vi "Measurement.vi"(0 "Position":T3(array[cluster]) {"Z" format="%.1f"; "Y" format="%.1f"; "X" format="%.1f"}, 1 "setup":T4=enum."Show Setup", 2 "Post Process":T2, 4 "File":T5, 5 "Results file":path, 7 "Raw data file":path, 11 "Setup filename":string) -> (14 "2nd plot":cluster{"X array":dbl[], "Y array":dbl[]}[](graph), 19 "Status Out":T1)   [LabVIEW 2015]
uses:
  Anemometry Sub Vis/Controls/Save_Data.ctl
  Anemometry Sub Vis/Controls/Setup.ctl
  Anemometry Sub Vis/Controls/Graph_Type.ctl
  Anemometry Sub Vis/Controls/Post_Process.ctl
  Anemometry Sub Vis/Gen Trav/Multi_Run_Status.ctl
  Anemometry Sub Vis/Controls/Inst_type.ctl
  ADAM Client/Sub VIs/ADAM Controls/Traverse_Level_State.ctl
  Anemometry Sub Vis/File/Setup_Filetype.ctl
  Anemometry Sub Vis/Globals/Meas_global.vi
  Anemometry Sub Vis/Globals/Trav_pos_global.vi
  Anemometry Sub Vis/Globals/Plug_in_data_global.vi
  Anemometry Sub Vis/Globals/Dynamic_call_global.ph.vi
  Anemometry Sub Vis/Globals/Preference_global.vi
  Anemometry Sub Vis/Globals/Constants_global.vi
  Anemometry Sub Vis/Globals/LDA_meas_global_2.vi
  Anemometry Sub Vis/Globals/LDA_meas_global_1.vi
  Anemometry Sub Vis/Acquisition/PWA/PWAtasksGLOBAL.vi
  Anemometry Sub Vis/Acquisition/Data_Translation/DataTranslation_global.vi
  Anemometry Sub Vis/Globals/Gas_management_global.vi
panel:
  in  "PP next block":bool
  out "Pause message":string
  out "Statistics":string[][](table)
  out "Actual Sampling freq":dbl=100.0 format="%.1f"
  in  "Desired Sampling freq (Hz)":dbl=100.0 format="%.1f"
  out "Current Block No":i32=5 caption="Current Block"
  in  "Pause":bool
  in  "No of Blocks":i32=5
  in  "stop":bool
  in  "No of samples":i32=1000 min=0 step=1
  in  "Tab Control":T6(tab)
  in  "Second Graph":T8={"Plot 1"=2, "Plot 2"=1, "Save graph"=0, "Plot Type"=enum."Vel histogram"} {"Save graph" items=["Do not save plot", "Save plot"]; "Plot 2" items=["Nothing", "mm"]; "Plot 1" items=["Nothing", "mm"]}
  in  "First Graph":T8={"Plot 1"=1, "Plot 2"=2, "Save graph"=0, "Plot Type"=enum."Velocity trace"} {"Save graph" items=["Do not save plot", "Save plot"]; "Plot 2" items=["Nothing", "mm"]; "Plot 1" items=["Nothing", "mm"]}
  out "First plot":cluster{"X array":dbl[], "Y array":dbl[]}[](graph)
  in  "Comments":string
  out "uv":dbl[][](graph)=[[-0.041806189081711534, -0.046435429052714985, -0.04035660097427599, -0.042187605126076694, -0.042052555599004206]]
  out "u^4":dbl[][](graph)
  out "u^3":dbl[][](graph)
  out "u^2":dbl[][](graph)=[[0.09743628875280319, 0.10575821456272283, 0.10126262927293661, 0.09890442087602569, 0.1022948212436432]]
  out "U":dbl[][](graph)=[[0.8295029456391334, 0.8915896983798417, 0.8415763502225625, 0.8394746126219594, 0.8466062785395404]]
  in  "Block average display control":cluster{"Name":string, "Include":bool}[](array[cluster])=[{"Name"="FF (C)", "Include"=FALSE}]
  in  "No of bins in histogram":i32=100
  out "Measurement time (min)":dbl=6.0 format="%.2f"
  in  "Correlate?":T9(ring)
  out "Diagnostic info":string[][](table)
  out "Array U":dbl[][](array[numeric]) format="%.2e"
  out "Array u^2":dbl[][](array[numeric]) format="%.2e"
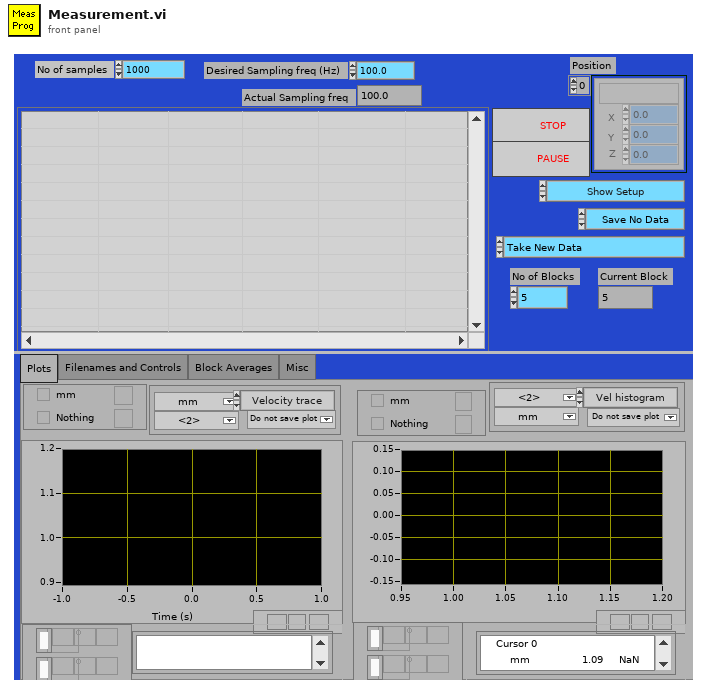
[diagram p1: front panel]
types:
  T1 = typedef "Multi_Run_Status.ctl" = enum16{"Continue", "Jump to Next Point", "Jump to Next Row", "Jump To Fall Back", "Terminate Run"}
  T2 = typedef "Post_Process.ctl" = enum16{"Take New Data", "Post Process Raw Data File"}
  T3 = cluster{"Name":string, "X":dbl, "Y":dbl, "Z":dbl}[]
  T4 = typedef "Setup.ctl" = enum16{"Run Program", "Show Setup", "Save Current Setup", "Setup Front Panel"}
  T5 = typedef "Save_Data.ctl" = enum16{"Save No Data", "Save Data"}
  T6 = enum32{"Plots", "Filenames and Controls", "Block Averages", "Misc"}
  T7 = typedef "Graph_Type.ctl" = enum16{"Show no graph", "Voltage trace", "Velocity trace", "Vel histogram", "Spectrum", "f.E(f) v Log f", "Auto-Corr"}
  T8 = cluster{"Plot 1":u16, "Plot 2":u16, "Save graph":u16, "Plot Type":T7}
  T9 = enum16{"Cross correlation off", "Show correlation panel", "Correlate without activating panel"}
  T10 = enum32{"Bad", "Idle", "Run top level", "Running"}
  T11 = cluster{"Name":string, "X":dbl, "Y":dbl, "Z":dbl}
  T12 = enum16{"Velocity", "Transit time", "Arrival time"}
  T13 = enum16{"Save no data", "Save data in new files", "Save data in existing files"}
  T14 = typedef "Inst_type.ctl" = enum16{"Propeller anemometer", "Raw voltage", "Pressure Transducer", "Pitot-static tube", "Preston tube", "Hot wire", "Cross wire 1", "Cross wire 2", "Generic Linear", "Generic Polynomial", "Generic BackPoly", "Fast FID", "Thermocouple", "Cold wire", "Pulsed Wire", "LDA Vel", "LDA Tran time", "LDA Arr time", "Microphone"}
  T15 = enum16{"Zero or one", "One", "Zero or more", "One or more"}
  T16 = cluster{"Weighting":dbl[], "Time (ms)":dbl[], "Voltage":dbl[], "Eng Values":dbl[]}
  T17 = typedef "Traverse_Level_State.ctl" = enum16{"Running", "Complete"}
  T18 = typedef "Setup_Filetype.ctl" = enum16{"Measurement Setups", "Calibration Setups", "General", "Results File Plotter Setups", "Speed Calib Tweaks"}
  T19 = typedef "Analysis_info_cluster.ctl" = cluster{"Colour":u32, "Inst type":T14, "Inst name":string, "Symbol":string, "Code name":string, "Extra Info":string, "Inst Array":T20, "Extra Titles":string[], "Extra Values":string[], "U":dbl, "u^2":dbl, "u^3":dbl, "u^4":dbl, "Skew_u":dbl, "Kurt_u":dbl, "Sd Error in Mean":dbl, "% u'/U":dbl, "X":dbl, "Y":dbl, "Z":dbl, "Timescale integral to 25%":dbl, "Sd Error in Variance":dbl, "Calib File":path, "Calib Constants":dbl[], "Output Position":bool, "Full Stats":bool, "Av Sampling Rate":dbl, "Av No of Samples":dbl, "Total Meas Time (s)":dbl, "ADAM Ch Name":string, "Max value":dbl, "Min value":dbl}
  T20 = typedef "Instrument_Array.ctl" = enum16{"PWA", "LDA", "Analogue"}
  T21 = typedef "LDA_Setup.ctl" = cluster{"dimensions":enum16{"1D", "2D"}, "Analogue Freq Multiplier":dbl}
  T22 = enum16{"Velocity", "Transit time", "Arrival time"}[]
  T23 = typedef "BSA_Type.ctl" = enum16{"57N11", "BSA F60"}
  T24 = typedef "BSA_info_Cluster.ctl" = cluster{"GPIB Address":string, "No of Check Bytes":i32, "Extra Info":string, "COLOUR":u32, "Wavelength (nm)":dbl}
  T25 = typedef "Ch_and_Spans.ctl" = cluster{"high limit (10V)":sgl, "low limit (-10V)":sgl, "Ch No":i16, "Var name":string, "Use Latest Calib":bool}
  T26 = cluster{"Weighting":dbl[], "Time (ms)":dbl[], "Voltage":dbl[], "Eng Values":dbl[]}[]
  T27 = cluster{"Insts for plotting[0]":u16, "Insts for plotting[1]":u16}
  T28 = typedef "PWA_Data.ctl" = enum16{"No PWA Data", "One Ch PWA"}
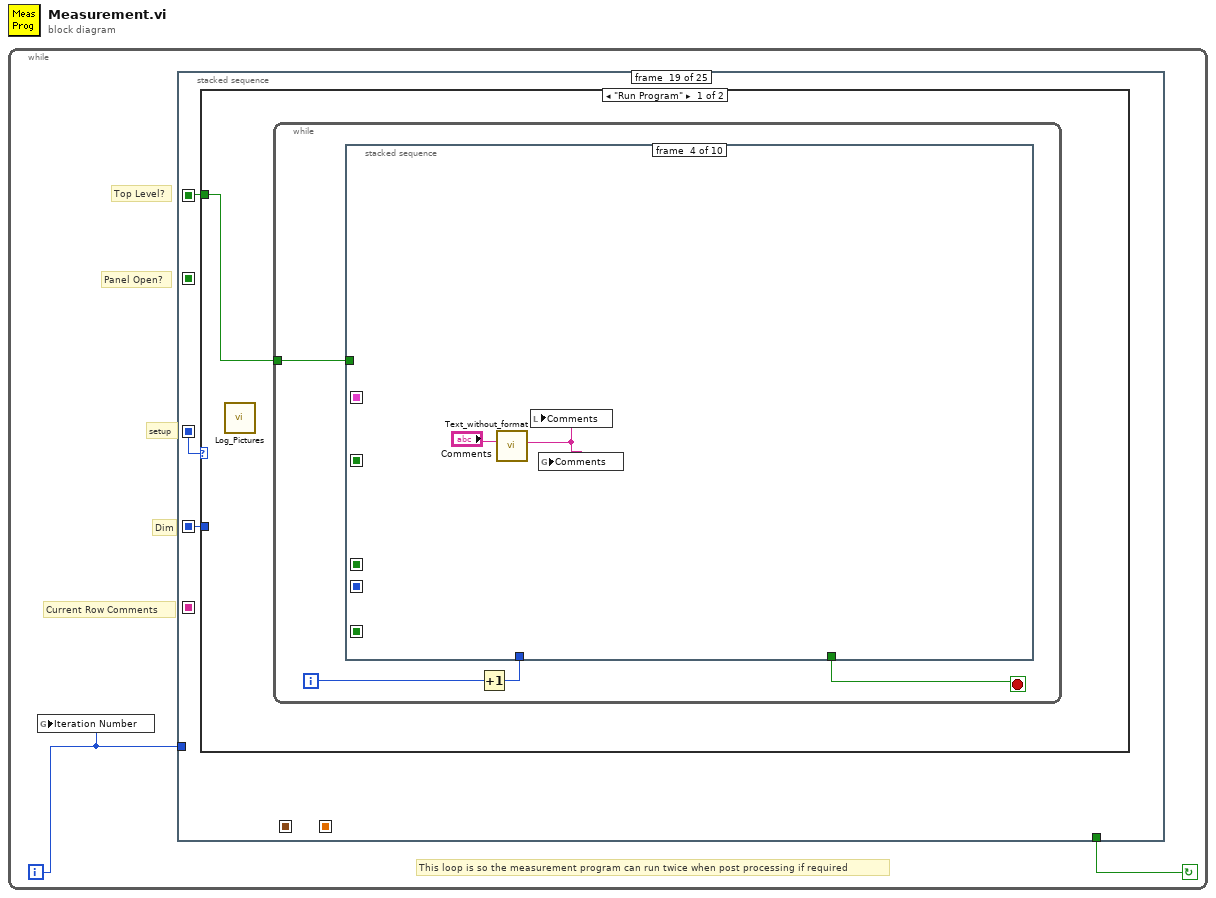
[diagram p0: block diagram]
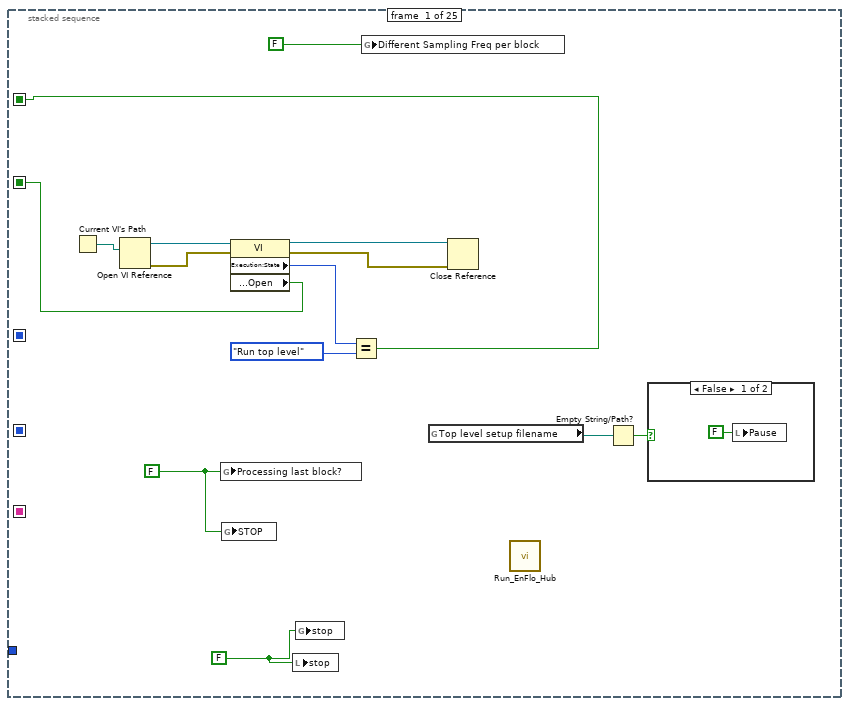
[diagram p2: hidden frame]
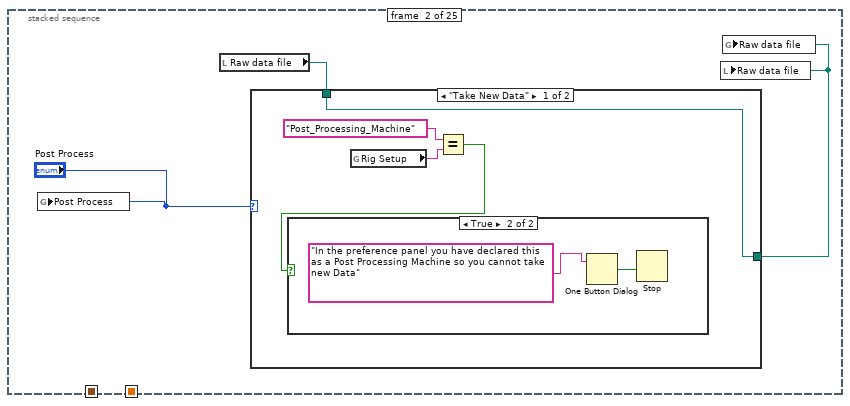
[diagram p4: hidden frame]
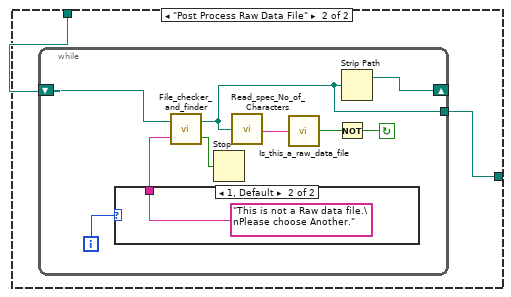
[diagram p6: hidden frame]
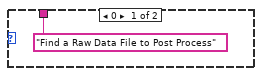
[diagram p7: hidden frame]
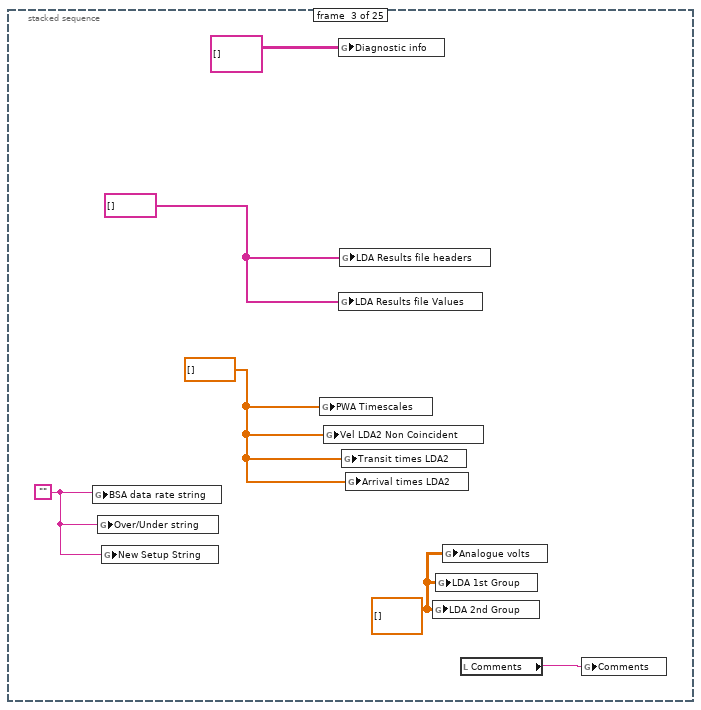
[diagram p8: hidden frame]
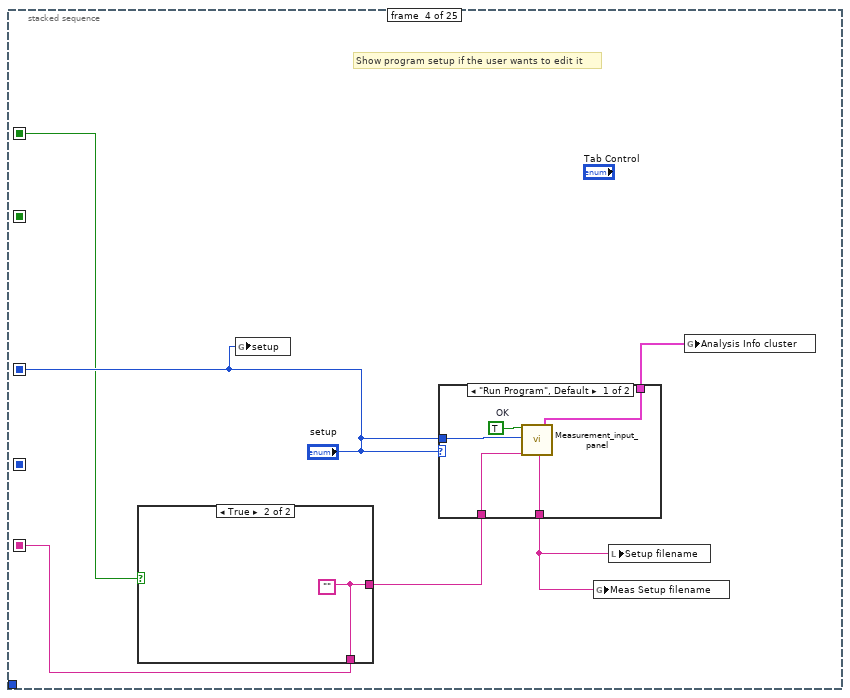
[diagram p9: hidden frame]
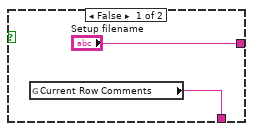
[diagram p10: hidden frame]
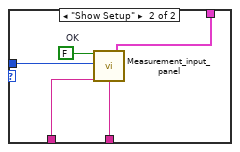
[diagram p11: hidden frame]
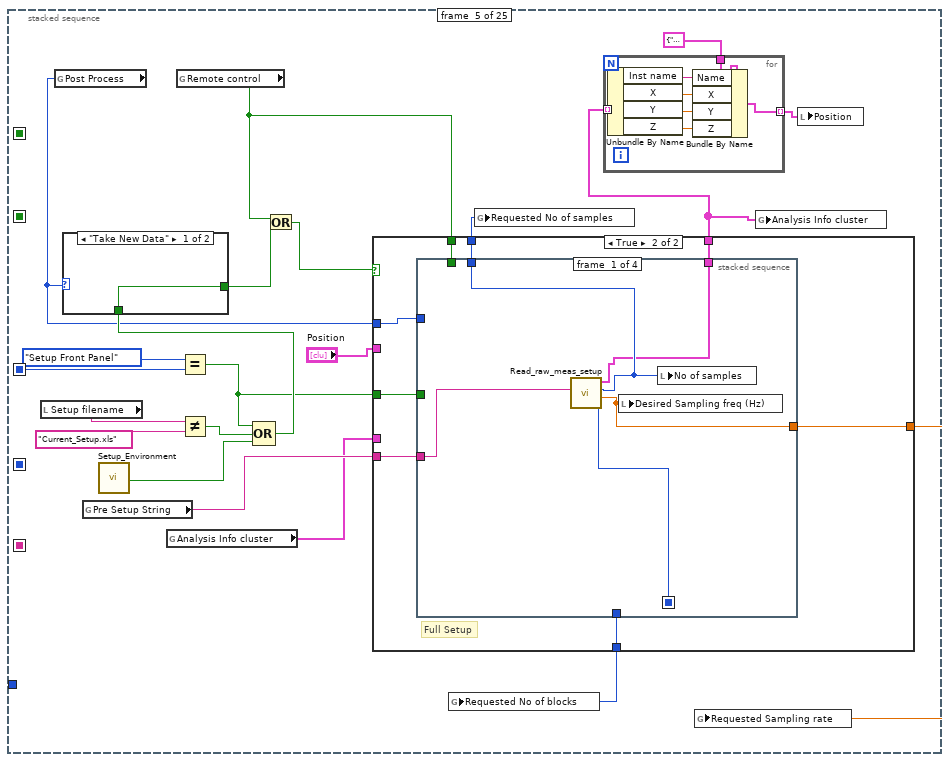
[diagram p12: hidden frame]
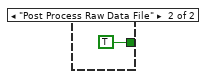
[diagram p13: hidden frame]
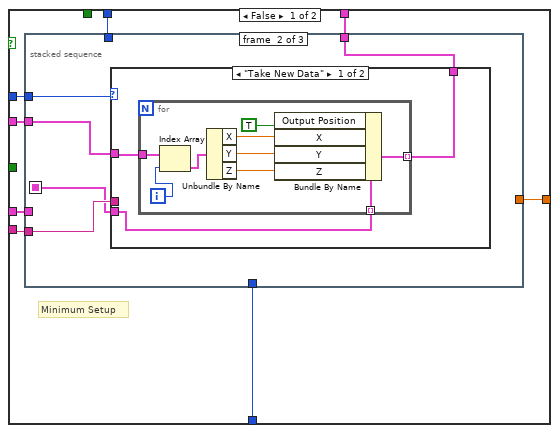
[diagram p14: hidden frame]
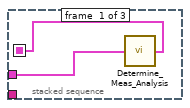
[diagram p15: hidden frame]
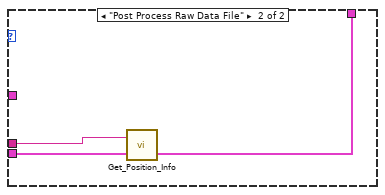
[diagram p16: hidden frame]
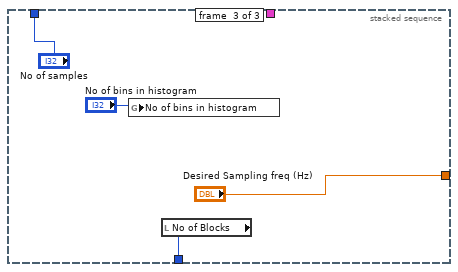
[diagram p17: hidden frame]
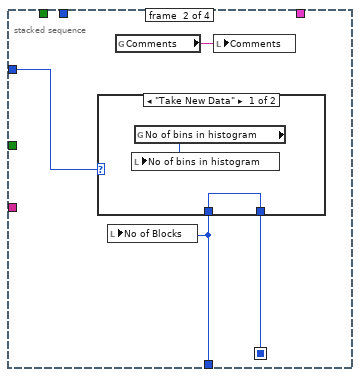
[diagram p18: hidden frame]
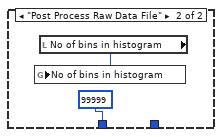
[diagram p19: hidden frame]
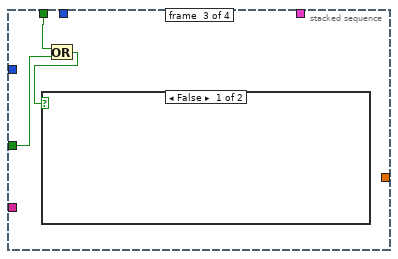
[diagram p20: hidden frame]
diagram:
  n1 = while {
    i -> [w1]
    stop <- w2 continue-if-true
    # "Current Row Comments"
    # "This loop is so the measurement program can run twice when post processing if required"
    # "Panel Open?"
    # "Top Level?"
    # "setup"
    # "Dim"
    n2 = global write "Meas_global.vi" "Iteration Number"(w1) -> ()
    n3 = stacked-sequence {
      seq-local: [_ _ _ _ _ _ _ _ w220 _ _ _ _ _ _ _ _ _ _ _ _ _ _ _ _] -> [_ _ _ _ _ _ _ _ _ _ _ _ _ _ _ _ _ _ w846 _ _ _ _ _ _]
      seq-local: [_ _ _ "setup" _ _ _ _ _ _ _ _ _ _ _ _ _ _ _ _ _ _ _ _ _] -> [_ _ _ _ w77 _ w184 _ w219 w308 _ _ _ _ w730 w749 w756 _ w847 w1047 w1097 w1167 _ _ w1288]
      seq-local: [_ _ _ _ _ _ _ _ _ _ _ _ _ _ _ _ w753 _ _ _ _ _ _ _ _] -> [_ _ _ _ _ _ _ _ _ _ _ _ _ _ _ _ _ _ _ w1037 _ _ _ _ _]
      seq-local: [w7 _ _ _ _ _ _ _ _ _ _ _ _ _ _ _ _ _ _ _ _ _ _ _ _] -> [_ _ _ w47 _ _ _ _ _ w288 _ _ _ _ w727 _ _ _ w845 _ _ _ _ _ _]
      seq-local: [w6 _ _ _ _ _ _ _ _ _ _ _ _ _ _ _ _ _ _ _ _ _ _ _ _] -> [_ _ _ _ _ _ _ _ _ _ _ _ w521 _ _ _ _ _ _ _ _ _ _ _ _]
      seq-local: [_ _ _ _ _ _ _ _ _ _ _ _ _ _ _ _ w751 _ _ _ _ _ _ _ _] -> [_ _ _ _ _ _ _ _ _ _ _ _ _ _ _ _ _ _ _ _ _ _ _ _ _]
      seq-local: [_ _ _ w46 _ _ _ _ _ _ _ _ _ _ _ _ _ _ _ _ _ _ _ _ _] -> [_ _ _ _ _ _ _ w215 _ _ _ _ _ _ _ _ _ _ _ _ _ _ _ w1251 _]
      tunnel: w1 -> [_ _ _ _ _ _ _ _ _ _ _ _ _ _ _ _ _ _ _ _ _ _ _ w1253 _]
      tunnel: [_ _ _ _ _ _ _ _ _ _ _ _ _ _ _ _ _ _ _ _ _ _ _ w1252 _] -> w2
      frame #0 {
        w15 = FALSE ("Processing last block?")
        w16 = FALSE ("stop")
        n4 = Current VI's Path() -> (path=w8:path)
        n5 = Open VI Reference(vi path=w8) -> (vi reference=w9:refnum<vi>, error out=w10:errorcluster)  [unwired: 1 in, 4 out]
        n6 = global write "Meas_global.vi" "Processing last block?"(w15) -> ()
        n7 = global write "PWAtasksGLOBAL.vi" "STOP"(w15) -> ()
        n8 = property class="VI"(reference=w9, error in=w10) -> (reference out=w11:refnum<vi>, error out=w12:errorcluster, "Execution:State"=w13:T10, "Front Panel.Open"=w6:bool)
        n9 = local write "stop"(w16) -> ()
        n10 = global write "Meas_global.vi" "stop"(w16) -> ()
        n11 = Equal?(x=w13, y=T10."Run top level" ("Exec.State")) -> (x = y?=w7:bool)
        n12 = global write "DataTranslation_global.vi" "Different Sampling Freq per block"(FALSE ("Different Sampling Freq per block")) -> ()
        n13 = global read "Trav_pos_global.vi" "Top level setup filename"() -> (w4:path)
        n14 = Close Reference(reference=w11, error in (no error)=w12) -> ()  [unwired: 1 out]
        n15 = call "Run_EnFlo_Hub.vi"() -> ()  [unwired: 1 in, 7 out]
        n16 = Empty String/Path?(string/path=w4) -> (empty?=w3:bool)
        n17 = case shown="False" w3 {
          frame False {
            n18 = local write "Pause"(FALSE ("Pause")) -> ()
          }
          frame True {
          }
        }
      }
      frame #1 {
        n19 = global write "Meas_global.vi" "Post Process"("Post Process") -> ()
        n20 = local read "Raw data file"() -> (w20:path)
        n21 = case shown="\"Take New Data\"" "Post Process" {
          tunnel: [w24 w28] -> w19
          tunnel: w20 -> [w24 w27]
          frame "Take New Data" {
            n22 = global read "Preference_global.vi" "Rig Setup"() -> (w23:string)
            n23 = Equal?(x="Post_Processing_Machine" ("Rig Setup"), y=w23) -> (x = y?=w21:bool)
            n24 = case shown="True" w21 {
              frame False {
              }
              frame True {
                n25 = One Button Dialog(message="In the preference panel you have declared this as a Post Processing Machine so you cannot take new Data") -> (true=w25:bool)  [unwired: 1 in]
                n26 = Stop(stop? (T)=w25) -> ()
              }
            }
          }
          frame "Post Process Raw Data File" {
            n27 = while {
              tunnel: [w30] -> w28
              shift-left: w27 -> [w32]
              shift-right: [w31] -> _
              i -> [w33]
              stop <- w34 continue-if-true
              n28 = case shown="1, Default" w33 {
                tunnel: ["Find a Raw Data File to Post Process" ("Promp if not found") "This is not a Raw data file.\nPlease choose Another." ("Promp if not found")] -> w37
                frame 0 {
                }
                frame 1, Default {
                }
              }
              n29 = call "File_checker_and_finder.vi"("Promp if not found"=w37, "Filename In"=w32) -> ("cancelled"=w29:bool, "Filename Out"=w30:path)
              n30 = Stop(stop? (T)=w29) -> ()
              n31 = call "Read_spec_No_of_Characters.vi"("Filename"=w30) -> ("character string"=w36:string)  [unwired: 1 out]
              n32 = call "Is_this_a_raw_data_file.vi"("character string"=w36) -> ("Raw Dat File?"=w35:bool)  [unwired: 2 out]
              n33 = Not(x=w35) -> (.not. x?=w34:bool)
              n34 = Strip Path(path=w30) -> (stripped path=w31:path)  [unwired: 1 out]
            }
          }
        }
        n35 = local write "Raw data file"(w19) -> ()
        n36 = global write "Meas_global.vi" "Raw data file"(w19) -> ()
      }
      frame #2 {
        w40 = dbl[][] [] ("LDA 2nd Group")
        w41 = dbl[] [] ("LDA Timescales")
        w43 = string[] [] ("Plug in values")
        w45 = ""
        n37 = global write "Meas_global.vi" "BSA data rate string"(w45) -> ()
        n38 = global write "Meas_global.vi" "Over/Under string"(w45) -> ()
        n39 = global write "Meas_global.vi" "New Setup String"(w45) -> ()
        n40 = global write "PWAtasksGLOBAL.vi" "PWA Timescales"(w41) -> ()
        n41 = global write "LDA_meas_global_2.vi" "Vel LDA2 Non Coincident"(w41) -> ()
        n42 = global write "Meas_global.vi" "Diagnostic info"(string[][] [] ("Diagnostic info")) -> ()
        n43 = global write "LDA_meas_global_1.vi" "LDA Results file Values"(w43) -> ()
        n44 = global write "LDA_meas_global_1.vi" "LDA Results file headers"(w43) -> ()
        n45 = global write "LDA_meas_global_2.vi" "Transit times LDA2"(w41) -> ()
        n46 = global write "LDA_meas_global_2.vi" "Arrival times LDA2"(w41) -> ()
        n47 = global write "LDA_meas_global_2.vi" "LDA 2nd Group"(w40) -> ()
        n48 = global write "LDA_meas_global_2.vi" "LDA 1st Group"(w40) -> ()
        n49 = global write "Meas_global.vi" "Analogue volts"(w40) -> ()
        n50 = local read "Comments"() -> (w44:string)
        n51 = global write "Meas_global.vi" "Comments"(w44) -> ()
      }
      frame #3 {
        # "Show program setup if the user wants to edit it"
        n52 = case shown="True" w47 {
          tunnel: ["Setup filename" w54] -> w50
          tunnel: [w52 w54] -> w46
          frame False {
            n53 = global read "Meas_global.vi" "Current Row Comments"() -> (w52:string)
          }
          frame True {
            w54 = ""
          }
        }
        n54 = global write "Meas_global.vi" "setup"("setup") -> ()
        n55 = case shown="\"Run Program\", Default" "setup" {
          tunnel: [w58 w63] -> w51
          tunnel: w50 -> [w57 w62]
          tunnel: [w56 w61] -> w49
          tunnel: "setup" -> [w55 w60]
          frame "Run Program", Default {
            w59 = TRUE  # OK
            n56 = call "Measurement_input_panel.vi"("OK"=w59, "setup"=w55, "Setup filename"=w57) -> ("Setup filename out"=w56:string, "Analysis Info cluster"=w58:T19[])  [unwired: 15 out]
          }
          frame "Show Setup" {
            w64 = FALSE  # OK
            n57 = call "Measurement_input_panel.vi"("OK"=w64, "setup"=w60, "Setup filename"=w62) -> ("Setup filename out"=w61:string, "Analysis Info cluster"=w63:T19[])  [unwired: 15 out]
          }
        }
        n58 = global write "Meas_global.vi" "Meas Setup filename"(w49) -> ()
        n59 = local write "Setup filename"(w49) -> ()
        n60 = global write "Meas_global.vi" "Analysis Info cluster"(w51) -> ()
      }
      frame #4 {
        n61 = local read "Setup filename"() -> (w81:string)
        n62 = global read "Meas_global.vi" "Post Process"() -> (w76:T2)
        n63 = global read "Meas_global.vi" "Pre Setup String"() -> (w72:string)
        n64 = call "Setup_Environment.vi"() -> ("First Time"=w73:bool)  [unwired: 1 in]
        n65 = global read "Meas_global.vi" "Analysis Info cluster"() -> (w69:T19[])
        n66 = global read "Meas_global.vi" "Remote control"() -> (w71:bool)
        n67 = Equal?(x=Setup."Setup Front Panel" ("setup"), y=w77) -> (x = y?=w70:bool)
        n68 = Not Equal?(x=w81, y="Current_Setup.xls" ("Setup filename")) -> (x != y?=w79:bool)
        n69 = Compound Arithmetic op=OR(w70, w79, w73) -> (w78:bool)
        n70 = case shown="\"Take New Data\"" w76 {
          tunnel: [w93 TRUE] -> w85
          tunnel: w78 -> [w93 _]
          frame "Take New Data" {
          }
          frame "Post Process Raw Data File" {
          }
        }
        n71 = Or(x=w71, y=w85) -> (x .or. y?=w84:bool)
        n72 = case shown="True" w84 {
          tunnel: w76 -> [w98 w136]
          tunnel: [w102 w135] -> w74
          tunnel: [w101 w130] -> w83
          tunnel: [w100 w134] -> w82
          tunnel: [w99 w133] -> w68
          tunnel: w72 -> [w97 w132]
          tunnel: "Position" -> [w96 _]
          tunnel: w71 -> [_ w131]
          tunnel: w70 -> [_ w129]
          tunnel: w69 -> [w95 _]
          frame False {
            # "Minimum Setup"
            n73 = stacked-sequence {
              seq-local: [w103 _ _] -> [_ w105 _]
              tunnel: [_ _ "Desired Sampling freq (Hz)"] -> w102
              tunnel: [_ _ w127] -> w101
              tunnel: [_ _ "No of samples"] -> w100
              tunnel: [_ w108 _] -> w99
              tunnel: w98 -> [_ w109 _]
              tunnel: w97 -> [_ w107 _]
              tunnel: w96 -> [_ w106 _]
              tunnel: w95 -> [w104 _ _]
              frame #0 {
                n74 = call "Determine_Meas_Analysis.vi"("Analysis info Cluster In"=w104) -> ("Analysis info Cluster Out"=w103:T19[])
              }
              frame #1 {
                n75 = case shown="\"Take New Data\"" w109 {
                  tunnel: [w110 w122] -> w108
                  tunnel: w106 -> [w112 _]
                  tunnel: w107 -> [_ w123]
                  tunnel: w105 -> [w111 w124]
                  frame "Take New Data" {
                    n76 = for {
                      tunnel: w112 -> [w115]
                      tunnel: w111 -> [w121] mode=indexing
                      tunnel: [w117] -> w110 mode=indexing
                      i -> [w116]
                      n77 = Index Array(array=w115, index=w116) -> (element=w114:T11)
                      n78 = Unbundle By Name(w114) -> ("X"=w118:dbl, "Y"=w119:dbl, "Z"=w120:dbl)
                      n79 = Bundle By Name(cluster=w121, "Output Position"=TRUE, "X"=w118, "Y"=w119, "Z"=w120) -> (w117:T19)
                    }
                  }
                  frame "Post Process Raw Data File" {
                    n80 = call "Get_Position_Info.vi"("Analysis Info cluster"=w124, "Setup file string"=w123) -> ("Analysis Info cluster 2"=w122:T19[])  [unwired: 1 in]
                  }
                }
              }
              frame #2 {
                n81 = global write "Meas_global.vi" "No of bins in histogram"("No of bins in histogram") -> ()
                n82 = local read "No of Blocks"() -> (w127:i32)
              }
            }
          }
          frame True {
            # "Full Setup"
            n83 = stacked-sequence {
              seq-local: [w138 _ _ _] -> [_ w143 _ _]
              tunnel: w136 -> [_ w144 _ w159]
              tunnel: [w141 _ _ _] -> w135
              tunnel: [w140 _ _ _] -> w134
              tunnel: [w137 _ _ _] -> w133
              tunnel: w132 -> [w139 _ _ _]
              tunnel: w131 -> [_ _ w152 _]
              tunnel: [_ w142 _ _] -> w130
              tunnel: w129 -> [_ _ w151 _]
              frame #0 {
                n84 = call "Read_raw_meas_setup.vi"("Setup file string"=w139) -> ("No of Blocks"=w138:i32, "Sampling freq (Hz)"=w141:dbl, "No of samples"=w140:i32, "Analysis Info cluster 2"=w137:T19[])  [unwired: 5 out]
                n85 = local write "Desired Sampling freq (Hz)"(w141) -> ()
                n86 = local write "No of samples"(w140) -> ()
              }
              frame #1 {
                n87 = case shown="\"Take New Data\"" w144 {
                  tunnel: [w147 99999 ("No of Blocks")] -> w142
                  tunnel: w143 -> [w147 _]
                  frame "Take New Data" {
                    n88 = global read "Meas_global.vi" "No of bins in histogram"() -> (w146:i32)
                    n89 = local write "No of bins in histogram"(w146) -> ()
                  }
                  frame "Post Process Raw Data File" {
                    n90 = local read "No of bins in histogram"() -> (w148:i32)
                    n91 = global write "Meas_global.vi" "No of bins in histogram"(w148) -> ()
                  }
                }
                n92 = local write "No of Blocks"(w142) -> ()
                n93 = global read "Meas_global.vi" "Comments"() -> (w145:string)
                n94 = local write "Comments"(w145) -> ()
              }
              frame #2 {
                n95 = Or(x=w152, y=w151) -> (x .or. y?=w150:bool)
                n96 = case shown="False" w150 {
                  frame False {
                  }
                  frame True {
                    n97 = global read "Meas_global.vi" "Pre Setup String"() -> (w153:string)
                    n98 = call "Get_Characters_from_string.vi"("Input string"=w153, "Variable name"="Results filename") -> ("Status"=w156:enum16{"Char in string", "Char not in string"}, "Value"=w155:string)  [unwired: 1 in]
                    n99 = case shown="\"Char in string\"" w156 {
                      tunnel: w155 -> [w158 _]
                      frame "Char in string" {
                        n100 = String To Path(string=w158) -> (path=w157:path)
                        n101 = local write "Results file"(w157) -> ()
                      }
                      frame "Char not in string" {
                      }
                    }
                  }
                }
              }
              frame #3 {
                n102 = case shown="\"Post Process Raw Data File\"" w159 {
                  frame "Take New Data" {
                    n103 = global read "Meas_global.vi" "Second Graph"() -> (w160:T8)
                    n104 = global read "Meas_global.vi" "First Graph"() -> (w161:T8)
                    n105 = local write "Second Graph"(w160) -> ()
                    n106 = local write "First Graph"(w161) -> ()
                  }
                  frame "Post Process Raw Data File" {
                  }
                }
              }
            }
          }
        }
        n107 = global write "Meas_global.vi" "Requested No of blocks"(w83) -> ()
        n108 = global write "Meas_global.vi" "Requested No of samples"(w82) -> ()
        n109 = for {
          tunnel: w68 -> [w92] mode=indexing
          tunnel: [w88] -> w66 mode=indexing
          tunnel: T11 {"Name"="", "X"=0.0, "Y"=0.0, "Z"=0.0} ("Position") -> [w87]
          n110 = Unbundle By Name(w92) -> ("Inst name"=w86:string, "X"=w89:dbl, "Y"=w90:dbl, "Z"=w91:dbl)
          n111 = Bundle By Name(cluster=w87, "Name"=w86, "X"=w89, "Y"=w90, "Z"=w91) -> (w88:T11)
        }
        n112 = global write "Meas_global.vi" "Requested Sampling rate"(w74) -> ()
        n113 = global write "Meas_global.vi" "Analysis Info cluster"(w68) -> ()
        n114 = local write "Position"(w66) -> ()
      }
      frame #5 {
        n115 = global read "Meas_global.vi" "Post Process"() -> (w162:T2)
        n116 = case shown="\"Post Process Raw Data File\"" w162 {
          tunnel: [w165 w166] -> w163
          frame "Take New Data" {
            n117 = Get Date/Time In Seconds() -> (seconds since 1Jan1904=w164:timestamp)
            n118 = To Double Precision Float(number=w164) -> (double precision float=w165:dbl)
          }
          frame "Post Process Raw Data File" {
            n119 = global read "Meas_global.vi" "Pre Setup String"() -> (w169:string)
            n120 = call "Get_Characters_from_string.vi"("Input string"=w169, "Variable name"="Seconds since 1/1/04") -> ("Value"=w167:string)  [unwired: 1 in, 1 out]
            n121 = call "String_2_Number.vi"("Value"=w167) -> ("Numeric"=w166:dbl)
          }
        }
        n122 = global write "Meas_global.vi" "Time Data was Aquired"(w163) -> ()
      }
      frame #6 {
        n123 = global read "Dynamic_call_global.ph.vi" "Initial Plug Ins"() -> (w189:string[])
        n124 = global read "Trav_pos_global.vi" "Source Control?"() -> (w186:bool)
        n125 = local read "Setup filename"() -> (w177:string)
        n126 = global read "Meas_global.vi" "Post Process"() -> (w175:T2)
        n127 = global read "Preference_global.vi" "Rig Setup"() -> (w172:string)
        n128 = Search 1D Array(1D array=w189, element="Puff_using_Arduino.vi") -> (index of element=w187:i32)  [unwired: 1 in]
        n129 = Equal?(x=w172, y="EnFlo_Tunnel") -> (x = y?=w170:bool)
        n130 = Equal?(x=w175, y=Post_Process."Take New Data" ("Post Process")) -> (x = y?=w173:bool)
        n131 = Equal?(x=Setup."Run Program" ("setup"), y=w184) -> (x = y?=w182:bool)
        n132 = Less Than 0?(x=w187) -> (x < 0?=w179:bool)
        n133 = Not Equal?(x=w177, y="Meas_FF_Bkgnd_Setup.xls") -> (x != y?=w181:bool)
        n134 = Not Equal?(x=w177, y="Auto_Calib_Setup.xls") -> (x != y?=w176:bool)
        n135 = Compound Arithmetic op=AND(w186, w182, w181, w176, w173, w170) -> (w180:bool)
        n136 = case shown="True" w180 {
          tunnel: w179 -> [_ w190]
          frame False {
          }
          frame True {
            n137 = global read "Gas_management_global.vi" "Source Live"() -> (w191:bool)
            n138 = Not(x=w191) -> (.not. x?=w192:bool)
            n139 = Select(t=w191, s=w190, f=w192) -> (s? t:f=w193:bool)
            n140 = global read "Preference_global.vi" "Default Source Establishment Time (s)"() -> (w194:dbl)
            n141 = case shown="False" w193 {
              tunnel: w194 -> [w196 w209]
              tunnel: w190 -> [w195 _]
              frame False {
                n142 = stacked-sequence {
                  tunnel: w196 -> [_ w205]
                  tunnel: w195 -> [w197 _]
                  frame #0 {
                    n143 = case shown="False" w197 {
                      tunnel: [w202 w204] -> w199
                      tunnel: [w201 w203] -> w198
                      frame True {
                        w201 = u32 0  # Time to hold source OFF (microseconds)
                        w202 = u32 1  # Time to hold source ON (microseconds)
                      }
                      frame False {
                        w203 = u32 1  # Time to hold source OFF (microseconds)
                        w204 = u32 0  # Time to hold source ON (microseconds)
                      }
                    }
                    n144 = call "Arduino_Timed_Release.vi"("Time to hold source ON (microseconds)"=w199, "Time to hold source OFF (microseconds)"=w198, "Number of cycles"=u16 1) -> ()  [unwired: 2 out]
                  }
                  frame #1 {
                    n145 = Greater Than 0?(x=w205) -> (x > 0?=w206:bool)
                    n146 = case shown="True" w206 {
                      tunnel: w205 -> [_ w207]
                      frame False {
                      }
                      frame True {
                        n147 = call "Wait_Seconds_with_display.vi"("Message"="Est Source", "Seconds to wait"=w207) -> ()  [unwired: 2 out]
                      }
                    }
                  }
                }
              }
              frame True {
                n148 = global read "Gas_management_global.vi" "Source Live Last changed"() -> (w213:timestamp)
                n149 = Get Date/Time In Seconds() -> (seconds since 1Jan1904=w214:timestamp)
                n150 = Subtract(x=w214, y=w213) -> (x-y=w212:dbl)
                n151 = Subtract(x=w209, y=w212) -> (x-y=w210:dbl)
                n152 = call "Wait_Seconds_with_display.vi"("Message"="Est Source", "Seconds to wait"=w210) -> ()  [unwired: 2 out]
              }
            }
          }
        }
      }
      frame #7 {
        n153 = local read "Comments"() -> (w218:string)
        n154 = Concatenate Strings(w215, w218) -> (w217:string)
        n155 = call "Text_without_format.vi"("Input string"=w217) -> ("Output string"=w216:string)
        n156 = local write "Comments"(w216) -> ()
        n157 = global write "Meas_global.vi" "Comments"(w216) -> ()
      }
      frame #8 {
        n158 = global read "Meas_global.vi" "LDA set up"() -> (w221:T21)
        n159 = Unbundle By Name(w221) -> ("dimensions"=w220:enum16{"1D", "2D"})
        n160 = global read "Meas_global.vi" "LDA data"() -> (w228:enum16{"No LDA data", "Take LDA data"})
        n161 = global read "Meas_global.vi" "Post Process"() -> (w230:T2)
        n162 = Equal?(x=w219, y=Setup."Show Setup" ("setup")) -> (x = y?=w222:bool)
        n163 = Equal?(x=w228, y=enum16{"No LDA data", "Take LDA data"}."Take LDA data" ("LDA data")) -> (x = y?=w224:bool)
        n164 = Equal?(x=w230, y=Post_Process."Take New Data" ("Post Process")) -> (x = y?=w225:bool)
        n165 = Compound Arithmetic op=AND(w224, w225) -> (w223:bool)
        n166 = case shown="True" w223 {
          tunnel: w220 -> [_ w239]
          tunnel: w219 -> [_ w238]
          tunnel: w222 -> [_ w236]
          frame False {
            n167 = Build Array(T12."Velocity", T12."Transit time", T12."Arrival time") -> (w231:T22)
            n168 = global write "LDA_meas_global_1.vi" "Number of measured quantities"(3 ("Number of measured quantities")) -> ()
            n169 = global write "LDA_meas_global_2.vi" "data type"(w231) -> ()
            n170 = global write "LDA_meas_global_1.vi" "data type"(w231) -> ()
          }
          frame True {
            n171 = global read "LDA_meas_global_1.vi" "BSA Type"() -> (w237:T23)
            n172 = case shown="\"BSA F60\"" w237 {
              tunnel: w239 -> [w241 _]
              tunnel: w238 -> [w240 _]
              tunnel: w236 -> [_ w277]
              frame "57N11" {
                n173 = stacked-sequence {
                  tunnel: w241 -> [w244 w270]
                  tunnel: w240 -> [w243 _]
                  frame #0 {
                    n174 = global read "Meas_global.vi" "Remote control"() -> (w242:bool)
                    n175 = case shown="\"1D\"" w244 {
                      tunnel: w243 -> [w246 w259]
                      tunnel: w242 -> [w245 w258]
                      frame "2D" {
                        n176 = while {
                          tunnel: w245 -> [w247]
                          tunnel: w246 -> [w248]
                          stop <- w249 continue-if-true
                          n177 = stacked-sequence {
                            tunnel: [_ _ w255] -> w249
                            tunnel: w248 -> [w250 w252 _]
                            tunnel: w247 -> [_ _ w254]
                            frame #0 {
                              w251 = "1"  # BSA Number
                              n178 = call "Control_BSA_setup.vi"("setup"=w250, "BSA number"=w251) -> ()  [unwired: 14 out]
                            }
                            frame #1 {
                              w253 = "2"  # BSA Number
                              n179 = call "Control_BSA_setup.vi"("setup"=w252, "BSA number"=w253) -> ()  [unwired: 14 out]
                            }
                            frame #2 {
                              n180 = case shown="False" w254 {
                                tunnel: [w256 FALSE ("ok")] -> w255
                                frame False {
                                n181 = call "BSA_setup_check.vi"() -> ("ok"=w256:bool)
                                }
                                frame True {
                                }
                              }
                            }
                          }
                        }
                      }
                      frame "1D" {
                        n182 = stacked-sequence {
                          tunnel: w259 -> [w260 _]
                          tunnel: w258 -> [_ _]
                          frame #0 {
                            w261 = "1"  # BSA Number
                            n183 = call "Control_BSA_setup.vi"("setup"=w260, "BSA number"=w261) -> ()  [unwired: 14 out]
                          }
                          frame #1 {
                            n184 = global read "LDA_meas_global_2.vi" "BSA2 info"() -> (w262:T24)
                            n185 = Unbundle By Name(w262) -> ("GPIB Address"=w263:string)
                            n186 = call "Set_BSA_Coincidence.vi"("GPIB address"=w263, "Set Coincidence"=enum16{"Slave", "Master", "Private"}."Slave") -> ()  [unwired: 1 in, 5 out]
                          }
                        }
                      }
                    }
                  }
                  frame #1 {
                    n187 = global read "Meas_global.vi" "Remote control"() -> (w268:bool)
                    n188 = Equal?(x=w270, y=enum16{"1D", "2D"}."2D" ("dimensions")) -> (x = y?=w266:bool)
                    n189 = Not(x=w268) -> (.not. x?=w267:bool)
                    n190 = And(x=w267, y=w266) -> (x .and. y?=w265:bool)
                    n191 = case shown="True" w265 {
                      frame False {
                      }
                      frame True {
                        n192 = global read "LDA_meas_global_1.vi" "BSA1 info"() -> (w272:T24)
                        n193 = global read "LDA_meas_global_2.vi" "BSA2 info"() -> (w273:T24)
                        n194 = Build Array(w272, w273) -> (w271:T24[])
                        n195 = for {
                          tunnel: w271 -> [w275] mode=indexing
                          n196 = Unbundle By Name(w275) -> ("GPIB Address"=w274:string)
                          n197 = call "Set_BSA_Coincidence.vi"("GPIB address"=w274, "Set Coincidence"=enum16{"Slave", "Master", "Private"}."Master") -> ()  [unwired: 1 in, 5 out]
                        }
                      }
                    }
                  }
                }
              }
              frame "BSA F60" {
                n198 = disable-structure shown="TARGET_TYPE==Windows" {
                  disable-tunnel: w277 -> [_ w278]
                  frame condition #0 {
                  }
                  frame condition #1 (active) {
                    n199 = while {
                      tunnel: w278 -> [w281]
                      stop <- w279 continue-if-true
                      n200 = call "Edit_BSA_IP.vi"("Show Panel"=w281) -> ("Run LDA Diagnostic Out"=w280:bool)  [unwired: 2 out]
                      n201 = case shown="True" w280 {
                        tunnel: [FALSE w283] -> w279
                        frame False {
                        }
                        frame True {
                          n202 = call "F60_Diagnostic.vi"() -> ("Edit BSA Setup Out"=w283:bool)  [unwired: 11 in]
                        }
                      }
                    }
                  }
                }
              }
            }
          }
        }
      }
      frame #9 {
        w293 = Save_Data."Save No Data" ("File")
        w309 = Post_Process."Take New Data"  # Post Process
        n203 = global read "Trav_pos_global.vi" "Meas Setup Number"() -> (w289:i32)
        n204 = Not Equal?(x=Setup."Run Program" ("setup"), y=w308) -> (x != y?=w294:bool)
        n205 = call "Current_Filepath.vi"("Short_Name"="Res" ("Data Type"), "Filename in"="Results file", "Data Type"="Results") -> ("Filename Out"=w287:path)  [unwired: 1 in, 1 out]
        n206 = global read "Meas_global.vi" "Remote control"() -> (w305:bool)
        n207 = global read "Meas_global.vi" "Post Process"() -> (w296:T2)
        n208 = Equal?(x="File", y=w293) -> (x = y?=w303:bool)
        n209 = case shown="1, Default" w289 {
          tunnel: [w312 w314] -> w290
          tunnel: w287 -> [w312 w321]
          tunnel: w289 -> [_ w322]
          frame 0 {
          }
          frame 1, Default {
            n210 = Add(x=96, y=w322) -> (x+y=w324:i32)
            n211 = Build Array(w324) -> (w325:i32[])
            n212 = Strip Path(path=w321) -> (stripped path=w315:path, name=w320:string)
            n213 = Byte Array To String(unsigned byte array=w325) -> (string=w318:string)
            n214 = call "Add_filename_suffix.vi"("Filename"=w320) -> ("Original Suffix"=w317:string, "Base name"=w319:string)  [unwired: 1 in, 2 out]
            n215 = Format Into String(format string="%s_%s%s", w319, w318, w317) -> (resulting string=w316:string)  [unwired: 2 in, 1 out]
            n216 = Build Path(base path=w315, name or relative path=w316) -> (appended path=w314:path)
          }
        }
        n217 = Equal?(x=w296, y=w309) -> (x = y?=w295:bool)
        n218 = And(x=w305, y=w295) -> (x .and. y?=w301:bool)
        n219 = Compound Arithmetic op=AND(w303, invert w305, w295, invert w294) -> (w304:bool)
        n220 = while {
          shift-left: _ -> [w330]
          shift-right: [w327] -> _
          tunnel: "File" -> [w328]
          tunnel: [w331] -> w302
          tunnel: w304 -> [w327]
          stop <- FALSE continue-if-true
          n221 = Compound Arithmetic op=AND(w327, invert w330) -> (w329:bool)
          n222 = case shown="False" w329 {
            tunnel: [w332 w335] -> w331
            tunnel: w328 -> [w332 _]
            frame False {
            }
            frame True {
              n223 = Two Button Dialog(message="Do you wish to save the data?", 1:"Save Data" ("F button name (\"Cancel\")"), 2:"Save No Data" ("T button name (\"OK\")")) -> (T button?=w336:bool)
              n224 = Select(t=Save_Data."Save No Data" ("File"), s=w336, f=Save_Data."Save Data" ("File")) -> (s? t:f=w335:T5)
            }
          }
        }
        n225 = Equal?(x=w293, y=w302) -> (x = y?=w292:bool)
        n226 = Or(x=w292, y=w294) -> (x .or. y?=w307:bool)
        n227 = case shown="False" w307 {
          tunnel: w290 -> [w351 w359]
          tunnel: [w350 w359] -> w310
          tunnel: "Raw data file" -> [w349 w360]
          tunnel: [w344 w360] -> w299
          tunnel: w308 -> [w348 _]
          tunnel: w302 -> [w347 _]
          tunnel: [w345 T13."Save no data" ("File output")] -> w297
          tunnel: [w346 w357] -> w291
          tunnel: w301 -> [_ w354]
          tunnel: w294 -> [_ w353]
          tunnel: w288 -> [w343 _]
          frame False {
            n228 = call "File_setup.vi"("Measurement is top level?"=w343, "Results file"=w351, "Raw data file"=w349, "setup"=w348, "File"=w347) -> ("Results file output"=w350:path, "Raw data file output"=w344:path, "Raw data option"=w346:enum16{"Save raw data", "Raw data not saved"}, "File output"=w345:T13)
          }
          frame True {
            w355 = enum16{"Save raw data", "Raw data not saved"}."Raw data not saved"  # Raw data option
            n229 = global read "Meas_global.vi" "Raw data option"() -> (w356:enum16{"Save raw data", "Raw data not saved"})
            n230 = Compound Arithmetic op=AND(w354, invert w353) -> (w352:bool)
            n231 = Select(t=w356, s=w352, f=w355) -> (s? t:f=w357:enum16{"Save raw data", "Raw data not saved"})
          }
        }
        n232 = case shown="\"Save raw data\"" w291 {
          tunnel: w299 -> [w340 w342]
          tunnel: [w340 w341] -> w298
          frame "Raw data not saved" {
          }
          frame "Save raw data" {
            n233 = call "Find_Unique_Filename.vi"("Path In"=w342) -> ("Unique Path Out"=w341:path)  [unwired: 1 in, 1 out]
          }
        }
        n234 = local write "Results file"(w310) -> ()
        n235 = global write "Meas_global.vi" "Results file"(w310) -> ()
        n236 = global write "Meas_global.vi" "Raw data option"(w291) -> ()
        n237 = global write "Meas_global.vi" "File"(w297) -> ()
        n238 = global write "Meas_global.vi" "Raw data file"(w298) -> ()
        n239 = local write "Raw data file"(w298) -> ()
        n240 = local write "File"(w302) -> ()
      }
      frame #10 {
        n241 = global read "Meas_global.vi" "Ch & spans"() -> (w363:T25[])
        n242 = local read "Block average display control"() -> (w366:cluster{"Name":string, "Include":bool}[])
        n243 = global read "Meas_global.vi" "LDA data"() -> (w361:enum16{"No LDA data", "Take LDA data"})
        n244 = global read "Meas_global.vi" "Analysis Info cluster"() -> (w362:T19[])
        n245 = global write "Meas_global.vi" "Ch & spans + mod limits"(w363) -> ()
        n246 = case shown="\"No LDA data\"" w361 {
          frame "No LDA data" {
          }
          frame "Take LDA data" {
            n247 = global write "Meas_global.vi" "Time Continuous Across Blocks"(FALSE ("Time Continuous Across Blocks")) -> ()
          }
        }
        n248 = for {
          tunnel: w362 -> [w375] mode=indexing
          tunnel: w366 -> [w374]
          tunnel: [w370] -> w365 mode=indexing
          tunnel: [w371] -> w364 mode=indexing
          i -> [w373]
          n249 = Unbundle By Name(w375) -> ("Symbol"=w370:string)
          n250 = Index Array(array=w374, index=w373) -> (element=w372:cluster{"Name":string, "Include":bool})
          n251 = Bundle By Name(cluster=w372, "Name"=w370) -> (w371:cluster{"Name":string, "Include":bool})
        }
        n252 = local write "Block average display control"(w364) -> ()
        n253 = Build Array (concatenate)("Nothing", w365) -> (w367:string[])
        n254 = property on="Plot 1" class="Ring (strict)"("Strings []"=w367) -> ()  [unwired: 2 in, 2 out]
        n255 = property on="Plot 1" class="Ring (strict)"("Strings []"=w367) -> ()  [unwired: 2 in, 2 out]
        n256 = property on="Plot 2" class="Ring (strict)"("Strings []"=w367) -> ()  [unwired: 2 in, 2 out]
        n257 = property on="Plot 2" class="Ring (strict)"("Strings []"=w367) -> ()  [unwired: 2 in, 2 out]
      }
      frame #11 {
        n258 = global read "Meas_global.vi" "Analysis Info cluster"() -> (w376:T19[])
        n259 = stacked-sequence {
          seq-local: [_ w404 _ _ _] -> [_ _ w435 w490 _]
          seq-local: [_ _ w436 _ _] -> [_ _ _ w489 _]
          seq-local: [_ w403 _ _ _] -> [_ _ w434 _ _]
          seq-local: [w382 _ _ _ _] -> [_ _ w432 _ _]
          seq-local: [w380 _ _ _ _] -> [_ _ w433 _ _]
          seq-local: [w378 _ _ _ _] -> [_ _ w431 _ _]
          tunnel: w376 -> [w385 w407 w437 _ w520]
          frame #0 {
            n260 = for {
              tunnel: w385 -> [w400] mode=indexing
              tunnel: [w399] -> w389
              stop <- w399 stop-if-true
              n261 = Unbundle By Name(w400) -> ("Inst type"=w401:T14)
              n262 = Equal?(x=w401, y=Inst_type."LDA Vel" ("Inst type")) -> (x = y?=w399:bool)
            }
            n263 = global read "Meas_global.vi" "Pre Setup String"() -> (w384:string)
            n264 = global read "Meas_global.vi" "Post Process"() -> (w386:T2)
            n265 = call "Correlation_Setup.vi"("Input string"=w384) -> ("Correlate"=w382:i32[][], "Error?"=w383:bool)
            n266 = Equal?(x=w386, y=Post_Process."Post Process Raw Data File" ("Post Process")) -> (x = y?=w388:bool)
            n267 = Compound Arithmetic op=AND(w389, w388, w383) -> (w380:bool)
            n268 = case shown="\"Correlate without activating panel\"" "Correlate?" {
              tunnel: w382 -> [w394 _ _]
              tunnel: [w392 FALSE FALSE] -> w381
              frame "Cross correlation off" {
                n269 = Array Size(array=w394) -> (size(s)=w396:i32[])
                n270 = Index Array(array=w396, index=0) -> (element=w393:i32)
                n271 = Greater Than 0?(x=w393) -> (x > 0?=w392:bool)
              }
              frame "Show correlation panel" {
              }
              frame "Correlate without activating panel" {
              }
            }
            n272 = Or(x=w381, y=w380) -> (x .or. y?=w379:bool)
            n273 = case shown="False" w379 {
              tunnel: [w390 w391] -> w378
              tunnel: "Correlate?" -> [w390 _]
              frame False {
              }
              frame True {
                w391 = T9."Correlate without activating panel" ("Correlate?")
                n274 = local write "Correlate?"(w391) -> ()
              }
            }
          }
          frame #1 {
            w405 = "RV (WT"
            n275 = String Length(string=w405) -> (length=w406:i32)
            n276 = for {
              tunnel: w407 -> [w426] mode=indexing
              shift-right: [w416] -> w408
              shift-left: i32[] [] -> [w417]
              tunnel: w406 -> [w414]
              tunnel: w405 -> [w412]
              tunnel: [w410] -> w403 mode=indexing
              i -> [w418]
              n277 = Unbundle By Name(w426) -> ("Inst name"=w410:string, "Symbol"=w425:string, "Code name"=w423:string)
              n278 = String Subset(string=w410, length (rest)=w414) -> (substring=w413:string)  [unwired: 1 in]
              n279 = Match Pattern(string=w423, regular expression="Derived") -> (offset past match=w422:i32)  [unwired: 1 in, 3 out]
              n280 = Not Equal?(x=w412, y=w413) -> (x != y?=w411:bool)
              n281 = Less Than 0?(x=w422) -> (x < 0?=w421:bool)
              n282 = Not Equal?(x="Sync", y=w425) -> (x != y?=w420:bool)
              n283 = Compound Arithmetic op=AND(w411, w420, w421) -> (w419:bool)
              n284 = case shown="True" w419 {
                tunnel: w418 -> [_ w430]
                tunnel: w417 -> [w427 w429]
                tunnel: [w427 w428] -> w416
                frame False {
                }
                frame True {
                  n285 = Build Array (concatenate)(w429, w430) -> (w428:i32[])
                }
              }
            }
            n286 = call "Chs_to_Correlate.vi"("Valid Ch to correlate"=w408) -> ("Correlation Pairs"=w404:i32[][])
          }
          frame #2 {
            n287 = case shown="False" w433 {
              tunnel: w437 -> [_ _]
              tunnel: [w440 w485] -> w436
              tunnel: w435 -> [w441 w485]
              tunnel: w434 -> [w445 _]
              tunnel: w432 -> [w439 _]
              tunnel: w431 -> [w438 _]
              frame False {
                n288 = for {
                  tunnel: w441 -> [w470] mode=indexing
                  tunnel: w445 -> [w475]
                  tunnel: [w466] -> w444 mode=indexing
                  tunnel: w439 -> [w471]
                  shift-right: [w467] -> w442
                  shift-left: string[] [] -> [w468]
                  n289 = Index Array(array=w470) -> (element #1=w477:i32, element #2=w476:i32)  [unwired: 2 in]
                  n290 = for {
                    tunnel: w470 -> [w484]
                    tunnel: w471 -> [w483] mode=indexing
                    tunnel: [w482] -> w469
                    stop <- w482 stop-if-true
                    n291 = Equal?(x=w484, y=w483) -> (x = y?=w482:bool)
                  }
                  n292 = Index Array(array=w475, index=w477) -> (element=w474:string)
                  n293 = Index Array(array=w475, index=w476) -> (element=w473:string)
                  n294 = Format Into String(format string="%s & %s", w474, w473) -> (resulting string=w466:string)  [unwired: 2 in, 1 out]
                  n295 = case shown="True" w469 {
                    tunnel: w468 -> [w478 w481]
                    tunnel: [w478 w480] -> w467
                    tunnel: w466 -> [_ w479]
                    frame False {
                    }
                    frame True {
                      n296 = Build Array (concatenate)(w481, w479) -> (w480:string[])
                    }
                  }
                }
                n297 = case shown="\"Show correlation panel\"" w438 {
                  tunnel: w444 -> [_ w453 w457]
                  tunnel: w442 -> [_ w451 w458]
                  tunnel: w441 -> [_ w449 w459]
                  tunnel: [i32[][] [] ("Correlation Pairs") w447 w460] -> w440
                  frame "Cross correlation off" {
                  }
                  frame "Show correlation panel" {
                    n298 = call "Select_Strings.vi"("Available Ch names"=w453, "Message"="Please select Channels to Correlate", "Selector mode"=T15."Zero or more", "Desired Ch names (in)"=w451) -> ("Ch Indicies Choosen"=w448:i32[])  [unwired: 2 in, 2 out]
                    n299 = for {
                      tunnel: w449 -> [w456]
                      tunnel: w448 -> [w455] mode=indexing
                      tunnel: [w454] -> w447 mode=indexing
                      n300 = Index Array(array=w456, index (row)=w455) -> (element=w454:i32[])  [unwired: 1 in]
                    }
                  }
                  frame "Correlate without activating panel" {
                    n301 = for {
                      tunnel: [w465] -> w460 mode=indexing
                      tunnel: w459 -> [w464]
                      tunnel: w458 -> [w463] mode=indexing
                      tunnel: w457 -> [w462]
                      n302 = Search 1D Array(1D array=w462, element=w463) -> (index of element=w461:i32)  [unwired: 1 in]
                      n303 = Index Array(array=w464, index (row)=w461) -> (element=w465:i32[])  [unwired: 1 in]
                    }
                  }
                }
              }
              frame True {
              }
            }
          }
          frame #3 {
            n304 = for {
              shift-right: [w497] -> w487
              shift-left: i32[][] [] -> [w498]
              tunnel: w490 -> [w499]
              tunnel: w489 -> [w496] mode=indexing
              n305 = for {
                tunnel: w499 -> [w514] mode=indexing
                tunnel: w496 -> [w513]
                tunnel: [w512] -> w495
                stop <- w512 stop-if-true
                n306 = Equal?(x=w513, y=w514) -> (x = y?=w512:bool)
              }
              n307 = case shown="True" w495 {
                tunnel: w498 -> [w500 w502]
                tunnel: w496 -> [_ w503]
                tunnel: [w500 w504] -> w497
                frame False {
                }
                frame True {
                  n308 = for {
                    tunnel: w503 -> [w507]
                    tunnel: w502 -> [w506] mode=indexing
                    tunnel: [w505] -> w501
                    stop <- w505 stop-if-true
                    n309 = Equal?(x=w507, y=w506) -> (x = y?=w505:bool)
                  }
                  n310 = case shown="False" w501 {
                    tunnel: w502 -> [w510 w511]
                    tunnel: w503 -> [w509 _]
                    tunnel: [w508 w511] -> w504
                    frame False {
                      n311 = Build Array (concatenate)(w510, w509) -> (w508:i32[][])
                    }
                    frame True {
                    }
                  }
                }
              }
            }
            n312 = global write "Meas_global.vi" "correlate"(w487) -> ()
            n313 = Array Size(array=w487) -> (size(s)=w494:i32[])
            n314 = Index Array(array=w494, index=0) -> (element=w491:i32)
            n315 = Equal To 0?(x=w491) -> (x = 0?=w492:bool)
            n316 = case shown="False" w492 {
              tunnel: [T9."Correlate without activating panel" ("Correlate?") T9."Cross correlation off" ("Correlate?")] -> w486
              frame False {
              }
              frame True {
              }
            }
            n317 = local write "Correlate?"(w486) -> ()
          }
          frame #4 {
            n318 = Array Size(array=w520) -> (size(s)=w518:i32)
            n319 = Initialize Array(T16 {"Weighting"=[], "Time (ms)"=[], "Voltage"=[], "Eng Values"=[]} ("Time Trace"), w518) -> (w517:T26)
            n320 = global write "Meas_global.vi" "Time Trace"(w517) -> ()
          }
        }
      }
      frame #12 {
        n321 = stacked-sequence {
          seq-local: [w527 _] -> [_ w549]
          tunnel: w521 -> [w526 _]
          frame #0 {
            n322 = call "LDA+_An_Analysis_mode.vi"("Second Graph"="Second Graph", "First Graph"="First Graph") -> ("Second Graph out"=w522:T8, "First Graph out"=w524:T8)  [unwired: 6 out]
            n323 = case shown="False" w526 {
              tunnel: [w537 w548] -> w525
              tunnel: w524 -> [w536 w548]
              tunnel: [w535 w547] -> w523
              tunnel: w522 -> [w534 w547]
              frame False {
                w532 = Graph_Type."Show no graph" ("Plot Type")
                n324 = Unbundle By Name(w536) -> ("Save graph"=w538:u16)
                n325 = Unbundle By Name(w534) -> ("Save graph"=w533:u16)
                n326 = case shown="0, Default" w538 {
                  tunnel: [w544 w546] -> w537
                  tunnel: w536 -> [w545 w546]
                  tunnel: w532 -> [w543 _]
                  frame 0, Default {
                    n327 = Bundle By Name(cluster=w545, "Plot Type"=w543) -> (w544:T8)
                  }
                  frame 1 {
                  }
                }
                n328 = case shown="0, Default" w533 {
                  tunnel: [w540 w542] -> w535
                  tunnel: w534 -> [w541 w542]
                  tunnel: w532 -> [w539 _]
                  frame 0, Default {
                    n329 = Bundle By Name(cluster=w541, "Plot Type"=w539) -> (w540:T8)
                  }
                  frame 1 {
                  }
                }
              }
              frame True {
              }
            }
            n330 = local write "Second Graph"(w523) -> ()
            n331 = local write "First Graph"(w525) -> ()
            n332 = global write "Meas_global.vi" "Second Graph"(w523) -> ()
            n333 = global write "Meas_global.vi" "First Graph"(w525) -> ()
            n334 = Unbundle By Name(w523) -> ("Plot Type"=w531:T7)
            n335 = Unbundle By Name(w525) -> ("Plot Type"=w530:T7)
            n336 = Build Array(w530, w531) -> (w527:T7[])
          }
          frame #1 {
            n337 = global read "Meas_global.vi" "Insts for plotting"() -> (w550:u16[][])
            n338 = while {
              tunnel: w550 -> [w557]
              tunnel: w549 -> [w556]
              shift-right: [w554] -> _
              shift-left: _ -> [w552]
              shift-right: [w553] -> _
              shift-left: _ -> [w551]
              stop <- TRUE stop-if-true
              n339 = for {
                tunnel: w557 -> [w563] mode=indexing
                tunnel: w556 -> [w562] mode=indexing
                tunnel: [w561] -> w554 mode=indexing
                tunnel: [w560] -> w553 mode=indexing
                tunnel: w552 -> [w559]
                tunnel: w551 -> [w558]
                i -> [w564]
                n340 = stacked-sequence {
                  seq-local: [w577 _] -> [_ w585]
                  seq-local: [w578 _] -> [_ w584]
                  seq-local: [w565 _] -> [_ w582]
                  tunnel: w564 -> [w574 w586]
                  tunnel: w563 -> [w569 _]
                  tunnel: w562 -> [w571 w583]
                  tunnel: [w569 _] -> w561
                  tunnel: [w571 _] -> w560
                  tunnel: w559 -> [w575 _]
                  tunnel: w558 -> [w573 _]
                  frame #0 {
                    n341 = property on="Plot 1" class="Ring (strict)"() -> ("Strings []"=w576:string[])  [unwired: 2 in, 2 out]
                    n342 = Array To Cluster(array=w569) -> (cluster=w581:T27)
                    n343 = Index Array(array=w575, index (row)=w574) -> (element=w570:u16[])  [unwired: 1 in]
                    n344 = Index Array(array=w573, index=w574) -> (element=w572:T7)
                    n345 = Unbundle(w581) -> ("Insts for plotting[0]"=w580:u16, "Insts for plotting[1]"=w579:u16)
                    n346 = Not Equal?(x=w572, y=w571) -> (x != y?=w568:bool)
                    n347 = Not Equal?(x=w569, y=w570) -> (x != y?=w567:bool[])
                    n348 = Index Array(array=w576, index=w580) -> (element=w577:string)
                    n349 = Index Array(array=w576, index=w579) -> (element=w578:string)
                    n350 = Or Array Elements(Boolean array=w567) -> (logical OR=w566:bool)
                    n351 = Or(x=w566, y=w568) -> (x .or. y?=w565:bool)
                  }
                  frame #1 {
                    n352 = case shown="True" w582 {
                      tunnel: w586 -> [_ w597]
                      tunnel: w585 -> [_ w594]
                      tunnel: w584 -> [_ w593]
                      tunnel: w583 -> [_ w589]
                      frame False {
                      }
                      frame True {
                        n353 = case shown="\"Velocity trace\"" w589 {
                          tunnel: [u8 0 u8 0 u8 0 u8 0 u8 0 u8 1 u8 0] -> w601
                          tunnel: [u8 0 u8 0 u8 0 u8 0 u8 1 u8 1 u8 0] -> w600
                          tunnel: [u8 0 u8 0 u8 0 u8 0 u8 1 u8 1 u8 0] -> w599
                          tunnel: [u8 0 u8 0 u8 0 u8 0 u8 1 u8 0 u8 0] -> w598
                          tunnel: [FALSE TRUE TRUE TRUE TRUE TRUE TRUE] -> w592
                          tunnel: [u8 0 u8 1 u8 1 u8 2 u8 0 u8 0 u8 2] -> w591
                          tunnel: [u8 0 u8 4 u8 1 u8 2 u8 0 u8 0 u8 1] -> w590
                          tunnel: ["" "Time (s)" "Time (s)" "" "" "" ""] -> w588
                          tunnel: ["" "Voltage" "Velocity" "" "" "" ""] -> w587
                          frame "Show no graph" {
                          }
                          frame "Voltage trace" {
                          }
                          frame "Velocity trace" {
                          }
                          frame "Vel histogram" {
                          }
                          frame "Spectrum" {
                          }
                          frame "f.E(f) v Log f" {
                          }
                          frame "Auto-Corr" {
                          }
                        }
                        n354 = case shown="1" w597 {
                          tunnel: w592 -> [w614 w627]
                          tunnel: w601 -> [w613 w626]
                          tunnel: w600 -> [w612 w625]
                          tunnel: w599 -> [w611 w624]
                          tunnel: w598 -> [w610 w623]
                          tunnel: u32 0 -> [w609 w622]
                          tunnel: u32 1 -> [w608 w620]
                          tunnel: w594 -> [w607 w621]
                          tunnel: w593 -> [w606 w619]
                          tunnel: w591 -> [w605 w618]
                          tunnel: w590 -> [w604 w617]
                          tunnel: w588 -> [w603 w616]
                          tunnel: w587 -> [w602 w615]
                          frame 0, Default {
                            n355 = property on="First plot" class="XYGraph (strict)"("Visible"=w614, "X Scale.Format & Precision:Format"=w613, "X Scale.Mapping Mode"=w612, "Y Scale.Format & Precision:Format"=w611, "Y Scale.Mapping Mode"=w610, "Active Plot"=w609, "Plot.Plot Name"=w607, "Active Plot"=w608, "Plot.Plot Name"=w606, "X Scale.Format & Precision:Precision"=w605, "Y Scale.Format & Precision:Precision"=w604, "XScale.NameLbl.Text"=w603, "YScale.NameLbl.Text"=w602) -> ()  [unwired: 2 in, 2 out]
                          }
                          frame 1 {
                            n356 = property on="2nd plot" class="XYGraph (strict)"("Visible"=w627, "X Scale.Format & Precision:Format"=w626, "X Scale.Mapping Mode"=w625, "Y Scale.Format & Precision:Format"=w624, "Y Scale.Mapping Mode"=w623, "Active Plot"=w622, "Plot.Plot Name"=w621, "Active Plot"=w620, "Plot.Plot Name"=w619, "X Scale.Format & Precision:Precision"=w618, "Y Scale.Format & Precision:Precision"=w617, "XScale.NameLbl.Text"=w616, "YScale.NameLbl.Text"=w615) -> ()  [unwired: 2 in, 2 out]
                          }
                        }
                      }
                    }
                  }
                }
              }
            }
          }
        }
      }
      frame #13 {
        n357 = local read "Second Graph"() -> (w702:T8)
        n358 = local read "First Graph"() -> (w701:T8)
        n359 = Unbundle By Name(w701) -> ("Plot 1"=w694:u16, "Plot 2"=w695:u16)
        n360 = Unbundle By Name(w702) -> ("Plot 1"=w696:u16, "Plot 2"=w697:u16)
        n361 = Build Array(w694, w695) -> (w698:u16[])
        n362 = Build Array(w696, w697) -> (w699:u16[])
        n363 = global read "Meas_global.vi" "Analysis Info cluster"() -> (w703:T19[])
        n364 = Decrement(x=w698) -> (x-1=w692:u16[])
        n365 = Decrement(x=w699) -> (x-1=w700:u16[])
        n366 = for {
          tunnel: w703 -> [w711]
          tunnel: w692 -> [w710] mode=indexing
          shift-right: [w704] -> _
          shift-left: u32 0 -> [w706]
          i -> [w705]
          n367 = Index Array(array=w711, index=w710) -> (element=w712:T19)
          n368 = Unbundle By Name(w712) -> ("Colour"=w707:u32)
          n369 = Equal?(x=w707, y=w706) -> (x = y?=w709:bool)
          n370 = Select(t=u32 13434624, s=w709, f=w707) -> (s? t:f=w704:u32)
          n371 = property on="First plot" class="XYGraph (strict)"("Active Plot"=w705, "Plot.Plot Color"=w704, "Plot.Fill/Point Color"=w704) -> ()  [unwired: 2 in, 2 out]
        }
        n372 = for {
          tunnel: w703 -> [w720]
          tunnel: w700 -> [w719] mode=indexing
          shift-right: [w715] -> _
          shift-left: u32 0 -> [w713]
          i -> [w718]
          n373 = Index Array(array=w720, index=w719) -> (element=w721:T19)
          n374 = Unbundle By Name(w721) -> ("Colour"=w714:u32)
          n375 = Equal?(x=w714, y=w713) -> (x = y?=w717:bool)
          n376 = Select(t=u32 13434624, s=w717, f=w714) -> (s? t:f=w715:u32)
          n377 = property on="2nd plot" class="XYGraph (strict)"("Active Plot"=w718, "Plot.Plot Color"=w715, "Plot.Fill/Point Color"=w715) -> ()  [unwired: 2 in, 2 out]
        }
      }
      frame #14 {
        n378 = global read "DataTranslation_global.vi" "Different Sampling Freq per block"() -> (w725:bool)
        n379 = global read "Meas_global.vi" "Remote control"() -> (w732:bool)
        n380 = global read "Meas_global.vi" "Post Process"() -> (w735:T2)
        n381 = global read "Meas_global.vi" "PWA Data"() -> (w726:T28)
        n382 = case shown="\"One Ch PWA\"" w726 {
          tunnel: [w736 w741] -> w728
          frame "No PWA Data" {
            n383 = local read "Desired Sampling freq (Hz)"() -> (w738:dbl)
            n384 = local read "No of samples"() -> (w737:i32)
            n385 = Divide(x=w737, y=w738) -> (x/y=w736:dbl)
          }
          frame "One Ch PWA" {
            n386 = local read "No of samples"() -> (w739:i32)
            n387 = global read "PWAtasksGLOBAL.vi" "PWA Freq. (Hz)"() -> (w740:dbl)
            n388 = global write "PWAtasksGLOBAL.vi" "PWA No. of Samples"(w739) -> ()
            n389 = Divide(x=w739, y=w740) -> (x/y=w741:dbl)
          }
        }
        n390 = Equal?(x=Setup."Run Program" ("setup"), y=w730) -> (x = y?=w723:bool)
        n391 = global read "Meas_global.vi" "Averaging time (min)"() -> (w731:dbl)
        n392 = Equal?(x=Post_Process."Take New Data" ("Post Process"), y=w735) -> (x = y?=w724:bool)
        n393 = And(x=w724, y=w723) -> (x .and. y?=w722:bool)
        n394 = Compound Arithmetic op=AND(invert w725, invert w727, invert w732, w722) -> (w733:bool)
        n395 = case shown="True" w733 {
          tunnel: w731 -> [_ w748]
          tunnel: w728 -> [_ w747]
          frame False {
          }
          frame True {
            n396 = Multiply(x=w748, y=60.0) -> (x*y=w744:dbl)
            n397 = Divide(x=w744, y=w747) -> (x/y=w743:dbl)
            n398 = Round Toward +Infinity(x=w743) -> (ceil(x): smallest int >= x=w742:dbl)
            n399 = To Long Integer(number=w742) -> (32bit integer=w746:i32)
            n400 = global write "Meas_global.vi" "Requested No of blocks"(w746) -> ()
            n401 = local write "No of Blocks"(w746) -> ()
          }
        }
      }
      frame #15 {
        n402 = case shown="\"Run Program\"" w749 {
          frame "Run Program" {
            n403 = call "Read_calibration_files.vi"() -> ()  [unwired: 1 out]
            n404 = global write "Meas_global.vi" "Repeat Measurement?"(FALSE ("Repeat Measurement?")) -> ()
          }
          frame "Show Setup", Default {
          }
        }
      }
      frame #16 {
        n405 = global read "Meas_global.vi" "Raw data option"() -> (w755:enum16{"Save raw data", "Raw data not saved"})
        n406 = Get Date/Time In Seconds() -> (seconds since 1Jan1904=w751:timestamp)
        n407 = To Double Precision Float(number=w751) -> (double precision float=w753:dbl)
        n408 = global read "Meas_global.vi" "Post Process"() -> (w754:T2)
        n409 = case shown="\"Setup Front Panel\"" w756 {
          tunnel: w755 -> [w758 _ _ _]
          tunnel: w754 -> [w757 _ w799 w808]
          frame "Run Program" {
            n410 = case shown="\"Take New Data\"" w757 {
              tunnel: w758 -> [w768 _]
              frame "Take New Data" {
                n411 = case shown="\"Raw data not saved\"" w768 {
                  frame "Save raw data" {
                  }
                  frame "Raw data not saved" {
                    w776 = FALSE  # Lock File
                    w773 = FALSE  # advisory dialog? (display:T)
                    w772 = FALSE  # append to file? (new file:F)
                    n412 = global read "Meas_global.vi" "Remote control"() -> (w774:bool)
                    n413 = call "Create_setup_string.vi"() -> ("Setup String"=w777:string)  [unwired: 1 out]
                    n414 = case shown="False" w774 {
                      tunnel: ["Current_Setup.xls" ("Setup filename") w779] -> w769
                      frame False {
                      }
                      frame True {
                        n415 = local read "Setup filename"() -> (w779:string)
                      }
                    }
                    n416 = call "Add_length_to_string.vi"("String in"=w777) -> ("String out"=w775:string)
                    n417 = call "Setup_Filepath.vi"("Setup File Type"=Setup_Filetype."Measurement Setups", "Filename in"=w769) -> ("Filename Out"=w770:path)  [unwired: 1 out]
                    n418 = call "Write_Characters_To_File.vi"("file path (dialog if empty)"=w770, "advisory dialog? (display:T)"=w773, "character string"=w775, "append to file? (new file:F)"=w772, "Lock File"=w776) -> ()  [unwired: 4 out]
                  }
                }
                n419 = global read "Meas_global.vi" "Requested No of samples"() -> (w762:i32)
                n420 = global read "Meas_global.vi" "Requested Sampling rate"() -> (w765:dbl)
                n421 = global read "Meas_global.vi" "Requested No of blocks"() -> (w761:i32)
                n422 = Divide(x=w762, y=w765) -> (x/y=w764:dbl)
                n423 = Multiply(x=w761, y=w764) -> (x*y=w760:dbl)
                n424 = Add(x=w760, y=120.0) -> (x+y=w759:dbl)
                n425 = call "Program_Active_Client.vi"("Mode"=enum16{"Program Active", "Traverse Level State"}."Program Active", "Time till next contact (Sec)"=w759, "Traverse level State"=Traverse_Level_State."Running") -> ()  [unwired: 3 out]
              }
              frame "Post Process Raw Data File" {
              }
            }
          }
          frame "Save Current Setup" {
            n426 = stacked-sequence {
              seq-local: [w782 _] -> [_ w785]
              seq-local: [w781 _] -> [_ w784]
              frame #0 {
                w783 = FALSE  # Save New File?
                n427 = call "Save_current_setup.vi"("Save New File?"=w783, "Setup File Type"=Setup_Filetype."Measurement Setups") -> ("Cancelled?"=w781:bool, "Saved filepath"=w782:path)  [unwired: 2 out]
              }
              frame #1 {
                n428 = case shown="False" w784 {
                  tunnel: w785 -> [w791 _]
                  frame False {
                    w788 = "Initial Probe positions" ("File Label")
                    w796 = FALSE  # append to file? (new file:F)
                    w797 = FALSE  # advisory dialog? (display:T)
                    w798 = FALSE  # Lock File
                    n429 = call "Input_Instrument_Positions.vi"("Filepath to Save"=w791) -> ("Output string"=w790:string)  [unwired: 1 out]
                    n430 = call "Create_setup_string.vi"() -> ("Setup String"=w789:string)  [unwired: 1 out]
                    n431 = call "Get_string_subset.vi"("String to split"=w790, "File Label"=w788) -> ("Output string"=w787:string)  [unwired: 2 in, 1 out]
                    n432 = call "Replace_data_in_Label_str.vi"("New data string"=w787, "Input string"=w789, "Variable name"=w788) -> ("Appended string"=w786:string)
                    n433 = call "Replace_data_in_setup_string.vi"("New data string"="", "Input string"=w786, "Variable name"="Comments") -> ("Appended string"=w792:string)
                    n434 = call "Add_length_to_string.vi"("String in"=w792) -> ("String out"=w795:string)
                    n435 = call "Write_Characters_To_File.vi"("file path (dialog if empty)"=w791, "advisory dialog? (display:T)"=w797, "character string"=w795, "append to file? (new file:F)"=w796, "Lock File"=w798) -> ()  [unwired: 4 out]
                  }
                  frame True {
                  }
                }
              }
            }
          }
          frame "Show Setup" {
            n436 = case shown="\"Take New Data\"" w799 {
              frame "Take New Data" {
                w804 = FALSE  # append to file? (new file:F)
                w805 = FALSE  # advisory dialog? (display:T)
                w806 = FALSE  # Lock File
                n437 = call "Create_setup_string.vi"() -> ("Setup String"=w807:string)  [unwired: 1 out]
                n438 = call "Add_length_to_string.vi"("String in"=w807) -> ("String out"=w803:string)
                n439 = call "Setup_Filepath.vi"("Setup File Type"=Setup_Filetype."Measurement Setups", "Filename in"="Current_Setup.xls" ("Setup filename")) -> ("Filename Out"=w801:path)  [unwired: 1 out]
                n440 = call "Write_Characters_To_File.vi"("file path (dialog if empty)"=w801, "advisory dialog? (display:T)"=w805, "character string"=w803, "append to file? (new file:F)"=w804, "Lock File"=w806) -> ()  [unwired: 4 out]
              }
              frame "Post Process Raw Data File" {
              }
            }
          }
          frame "Setup Front Panel" {
            n441 = case shown="\"Take New Data\"" w808 {
              frame "Take New Data" {
                w813 = FALSE  # append to file? (new file:F)
                w814 = FALSE  # advisory dialog? (display:T)
                w815 = FALSE  # Lock File
                n442 = call "Create_setup_string.vi"() -> ("Setup String"=w816:string)  [unwired: 1 out]
                n443 = call "Add_length_to_string.vi"("String in"=w816) -> ("String out"=w812:string)
                n444 = call "Setup_Filepath.vi"("Setup File Type"=Setup_Filetype."Measurement Setups", "Filename in"="Current_Setup.xls" ("Setup filename")) -> ("Filename Out"=w810:path)  [unwired: 1 out]
                n445 = call "Write_Characters_To_File.vi"("file path (dialog if empty)"=w810, "advisory dialog? (display:T)"=w814, "character string"=w812, "append to file? (new file:F)"=w813, "Lock File"=w815) -> ()  [unwired: 4 out]
              }
              frame "Post Process Raw Data File" {
              }
            }
          }
        }
        n446 = global write "Meas_global.vi" "Actual Measurement time (min)"(0.0 ("Max Measurement time (min)")) -> ()
      }
      frame #17 {
        n447 = global read "Dynamic_call_global.ph.vi" "Initial Plug Ins"() -> (w818:string[])
        n448 = global read "Dynamic_call_global.ph.vi" "Initial Plug Ins Extra"() -> (w819:string[])
        n449 = Build Array (concatenate)(w819, w818) -> (w817:string[])
        n450 = Array Size(array=w817) -> (size(s)=w821:i32)
        n451 = Greater Than 0?(x=w821) -> (x > 0?=w820:bool)
        n452 = case shown="True" w820 {
          tunnel: w817 -> [_ w822]
          frame False {
          }
          frame True {
            n453 = stacked-sequence {
              tunnel: w822 -> [w824 _]
              frame #0 {
                n454 = global read "Meas_global.vi" "Post Process"() -> (w826:T2)
                n455 = call "Plug_in_Directories.vi"() -> ("Initial"=w823:path)  [unwired: 3 out]
                n456 = Equal?(x=w826, y=Post_Process."Post Process Raw Data File" ("Post Process")) -> (x = y?=w825:bool)
                n457 = for {
                  tunnel: w825 -> [w832]
                  tunnel: w824 -> [w829] mode=indexing
                  tunnel: w823 -> [w828]
                  w839 = FALSE  # Dialog Box (T)
                  n458 = Build Path(base path=w828, name or relative path=w829) -> (appended path=w830:path)
                  n459 = Open VI Reference(vi path=w830) -> (vi reference=w837:refnum<vi>, error out=w836:errorcluster)  [unwired: 2 in, 3 out]
                  n460 = property class="VI"(reference=w837, error in=w836, "Front Panel Window:Open"=TRUE ("Wait until done")) -> (reference out=w835:refnum<vi>, error out=w834:errorcluster)
                  n461 = invoke class="VI" method="Run VI"(reference=w835, error in=w834, "Wait until done"=w832, "Auto Dispose Ref"=FALSE) -> (reference out=w842:refnum<vi>, error out=w841:errorcluster)  [unwired: 1 in, 3 out]
                  n462 = Close Reference(reference=w842, error in (no error)=w841) -> (error out=w840:errorcluster)
                  n463 = call "EnFlo_Error_Handler.vi"("error in (no error)"=w840, "Error Type"="Launching Initial Plug In", "Dialog Box (T)"=w839) -> ()  [unwired: 3 out]
                }
              }
              frame #1 {
                n464 = global read "Meas_global.vi" "Requested No of blocks"() -> (w844:i32)
                n465 = global read "Meas_global.vi" "Comments"() -> (w843:string)
                n466 = local write "Comments"(w843) -> ()
                n467 = local write "No of Blocks"(w844) -> ()
              }
            }
          }
        }
      }
      frame #18 {
        n468 = case shown="\"Run Program\"" w847 {
          tunnel: w845 -> [w848 _]
          tunnel: w846 -> [_ w941]
          frame "Run Program" {
            n469 = call "Log_Pictures.vi"() -> ()  [unwired: 12 in]
            n470 = while {
              tunnel: w848 -> [w849]
              i -> [w850]
              stop <- w851 stop-if-true
              n471 = Increment(x=w850) -> (x+1=w852:i32)
              n472 = stacked-sequence {
                seq-local: [_ _ _ _ _ "Block average display control" _ _ _ _] -> [_ _ _ _ _ _ w886 _ _ _]
                seq-local: [_ _ _ _ _ _ w884 _ _ _] -> [_ _ _ _ _ _ _ w902 _ _]
                seq-local: [_ _ _ _ w867 _ _ _ _ _] -> [_ _ _ _ _ _ _ _ _ w934]
                seq-local: [_ w855 _ _ _ _ _ _ _ _] -> [_ _ w861 _ _ _ _ _ _ _]
                seq-local: [_ _ w859 _ _ _ _ _ _ _] -> [_ _ _ _ _ _ _ _ _ w937]
                tunnel: w852 -> [w853 _ w860 _ _ w876 _ _ _ w938]
                tunnel: [_ _ w859 _ _ _ _ _ _ _] -> w851
                tunnel: w849 -> [_ _ _ _ w866 _ _ _ _ _]
                frame #0 {
                  w854 = string[] [] ("Plug in titles")
                  n473 = global write "Meas_global.vi" "Current Block No"(w853) -> ()
                  n474 = global write "Dynamic_call_global.ph.vi" "Plug in titles"(w854) -> ()
                  n475 = global write "Dynamic_call_global.ph.vi" "Plug in values"(w854) -> ()
                  "Current Block No" <- w853
                }
                frame #1 {
                  n476 = call "Get_data.vi"() -> ("EOF? and Error status"=w855:bool, "Block Header"=w856:string)  [unwired: 10 out]
                  n477 = global write "Plug_in_data_global.vi" "Block Header"(w856) -> ()
                }
                frame #2 {
                  n478 = property on="No of Blocks" class="DigNum (strict)"() -> ("ControlIndex"=w857:i32)  [unwired: 2 in, 2 out]
                  n479 = global write "Meas_global.vi" "Requested No of blocks"("No of Blocks") -> ()
                  n480 = Less Or Equal?(x="No of Blocks", y=w860) -> (x <= y?=w862:bool)
                  n481 = global write "Meas_global.vi" "Nblocks Index"(w857) -> ()
                  n482 = Compound Arithmetic op=OR(w861, w862) -> (w859:bool)
                  n483 = case shown="True" w859 {
                    tunnel: w860 -> [_ w863]
                    frame False {
                    }
                    frame True {
                      n484 = global write "Meas_global.vi" "Requested No of blocks"(w863) -> ()
                      n485 = local write "No of Blocks"(w863) -> ()
                    }
                  }
                  n486 = global write "Meas_global.vi" "Processing last block?"(w859) -> ()
                  n487 = global write "PWAtasksGLOBAL.vi" "STOP"(w859) -> ()
                }
                frame #3 {
                  n488 = call "Text_without_format.vi"("Input string"="Comments") -> ("Output string"=w864:string)
                  n489 = local write "Comments"(w864) -> ()
                  n490 = global write "Meas_global.vi" "Comments"(w864) -> ()
                }
                frame #4 {
                  n491 = call "Process_data.vi"("Measurement top level?"=w866) -> ("Vel stat display"=→"Statistics":string[][], "First Plot data Cluster"=→"First plot":cluster{"X array":dbl[], "Y array":dbl[]}[], "Second Plot Data Cluster"=→"2nd plot":cluster{"X array":dbl[], "Y array":dbl[]}[], "Max Measurement time up"=w867:bool)  [unwired: 5 in]
                }
                frame #5 {
                  n492 = global read "Meas_global.vi" "Actual Measurement time (min)"() -> (→"Measurement time (min)":dbl)
                  n493 = global read "Meas_global.vi" "Actual Sampling rate (Hz)"() -> (→"Actual Sampling freq":dbl)
                  n494 = call "Display_blocks.vi"("Block No"=w876, "Block average display"="Block average display control") -> ("u^4"=→"u^4":dbl[][], "u^3"=→"u^3":dbl[][], "uv"=→"uv":dbl[][], "u^2"=→"u^2" →"Array u^2":dbl[][], "U"=→"U" →"Array U":dbl[][])  [unwired: 4 out]
                }
                frame #6 {
                  n495 = global read "Meas_global.vi" "Analysis Info cluster"() -> (w885:T19[])
                  n496 = global read "Meas_global.vi" "Diagnostic info"() -> (w883:string[][])
                  n497 = for {
                    tunnel: w886 -> [w901] mode=indexing
                    tunnel: w885 -> [w898] mode=indexing
                    tunnel: [w900] -> w884 mode=indexing if=w899
                    tunnel: [w888] -> w882 mode=indexing
                    tunnel: [w887] -> w881 mode=indexing
                    n498 = Unbundle By Name(w898) -> ("Colour"=w900:u32)
                    n499 = Unbundle By Name(w901) -> ("Include"=w899:bool)
                    n500 = Unbundle By Name(w898) -> ("Inst name"=w892:string, "Av Sampling Rate"=w894:dbl, "Av No of Samples"=w891:dbl)
                    n501 = Format Into String(format string="%s Freq Hz", w892) -> (resulting string=w896:string)  [unwired: 2 in, 1 out]
                    n502 = Format Into String(format string="%s Samples per block", w892) -> (resulting string=w889:string)  [unwired: 2 in, 1 out]
                    n503 = Number To Decimal String(number=w894) -> (decimal integer string=w895:string)  [unwired: 1 in]
                    n504 = Number To Decimal String(number=w891) -> (decimal integer string=w890:string)  [unwired: 1 in]
                    n505 = Build Array(w896, w895) -> (w888:string[])
                    n506 = Build Array(w889, w890) -> (w887:string[])
                  }
                  n507 = Build Array (concatenate)(w883, w882, w881) -> (→"Diagnostic info":string[][])
                }
                frame #7 {
                  n508 = for {
                    tunnel: w902 -> [w903] mode=indexing
                    i -> [w904]
                    n509 = property on="U" class="WFGraph (strict)"("Active Plot"=w904, "Plot.Plot Color"=w903, "Plot.Fill/Point Color"=w903) -> ()  [unwired: 2 in, 2 out]
                    n510 = property on="u^3" class="WFGraph (strict)"("Active Plot"=w904, "Plot.Plot Color"=w903, "Plot.Fill/Point Color"=w903) -> ()  [unwired: 2 in, 2 out]
                    n511 = property on="u^4" class="WFGraph (strict)"("Active Plot"=w904, "Plot.Plot Color"=w903, "Plot.Fill/Point Color"=w903) -> ()  [unwired: 2 in, 2 out]
                    n512 = property on="u^2" class="WFGraph (strict)"("Active Plot"=w904, "Plot.Plot Color"=w903, "Plot.Fill/Point Color"=w903) -> ()  [unwired: 2 in, 2 out]
                  }
                }
                frame #8 {
                  n513 = case shown="True" "Pause" {
                    frame False {
                    }
                    frame True {
                      n514 = global read "Meas_global.vi" "Post Process"() -> (w906:T2)
                      n515 = case shown="\"Post Process Raw Data File\"" w906 {
                        frame "Take New Data" {
                          n516 = call "Program_Active_Client.vi"("Mode"=enum16{"Program Active", "Traverse Level State"}."Program Active", "Time till next contact (Sec)"=12000.0, "Traverse level State"=Traverse_Level_State."Running") -> ()  [unwired: 3 out]
                          n517 = while {
                            i -> [w913]
                            stop <- w914 continue-if-true
                            n518 = Quotient & Remainder(x=w913, y=10) -> (x-y*floor(x/y)=w911:i32)  [unwired: 1 out]
                            n519 = Equal To 0?(x=w911) -> (x = 0?=w910:bool)
                            n520 = stacked-sequence {
                              seq-local: [_ w916 _ _] -> [_ _ w918 _]
                              tunnel: [_ w916 _ _] -> w914
                              tunnel: w910 -> [_ _ _ w920]
                              frame #0 {
                                "Pause message" <- "Measurement Program Paused!!!!" ("Pause message")
                              }
                              frame #1 {
                                n521 = global write "Trav_pos_global.vi" "Paused During Row?"(TRUE ("Paused During Row?")) -> ()
                                n522 = local read "Pause"() -> (w916:bool)
                              }
                              frame #2 {
                                n523 = property on="Pause message" class="Str"("Blinking"=w918, "Visible"=w918) -> ()  [unwired: 2 in, 2 out]
                                n524 = Wait Until Next ms Multiple(millisecond multiple=u32 1000) -> ()  [unwired: 1 out]
                              }
                              frame #3 {
                                n525 = case shown="False" w920 {
                                frame False {
                                }
                                frame True {
                                n526 = Current VI's Path() -> (path=w921:path)
                                n527 = call "Bring_to_front.vi"("path"=w921) -> ()
                                }
                                }
                              }
                            }
                          }
                        }
                        frame "Post Process Raw Data File" {
                          n528 = stacked-sequence {
                            seq-local: [_ w924 _ _] -> [_ _ _ w931]
                            frame #0 {
                              n529 = property on="PP next block" class="Bool (strict)"("Visible"=TRUE) -> ()  [unwired: 2 in, 2 out]
                              n530 = local write "PP next block"(FALSE ("PP next block")) -> ()
                            }
                            frame #1 {
                              n531 = while {
                                tunnel: [w928] -> w924
                                stop <- w925 stop-if-true
                                n532 = local read "stop"() -> (w928:bool)
                                n533 = local read "Pause"() -> (w926:bool)
                                n534 = Compound Arithmetic op=OR(w928, "PP next block", invert w926) -> (w925:bool)
                                n535 = case shown="False" w925 {
                                frame False {
                                n536 = Wait (ms)(milliseconds to wait=u32 200) -> ()  [unwired: 1 out]
                                }
                                frame True {
                                }
                                }
                              }
                            }
                            frame #2 {
                              n537 = property on="PP next block" class="Bool (strict)"("Visible"=FALSE) -> ()  [unwired: 2 in, 2 out]
                            }
                            frame #3 {
                              n538 = Stop(stop? (T)=w931) -> ()
                            }
                          }
                        }
                      }
                    }
                  }
                }
                frame #9 {
                  n539 = global read "Meas_global.vi" "stop"() -> (w932:bool)
                  n540 = Compound Arithmetic op=OR("stop", w934, w932) -> (w933:bool)
                  n541 = Compound Arithmetic op=AND(w933, invert w937) -> (w936:bool)
                  n542 = case shown="True" w936 {
                    tunnel: w938 -> [_ w940]
                    frame False {
                    }
                    frame True {
                      n543 = Increment(x=w940) -> (x+1=w939:i32)
                      n544 = local write "No of Blocks"(w939) -> ()
                      n545 = global write "Meas_global.vi" "Requested No of blocks"(w939) -> ()
                    }
                  }
                }
              }
            }
          }
          frame Default {
            n546 = stacked-sequence {
              seq-local: [w942 _ _ _ _ _ _] -> [_ _ _ _ _ w1016 _]
              seq-local: [_ w948 _ _ _ _ _] -> [_ _ _ _ _ w1015 _]
              seq-local: [_ _ _ w979 _ _ _] -> [_ _ _ _ _ w1014 _]
              seq-local: [_ _ _ _ w992 _ _] -> [_ _ _ _ _ w1012 _]
              seq-local: [_ w947 _ _ _ _ _] -> [_ _ _ _ _ _ w1025]
              seq-local: [_ _ w973 _ _ _ _] -> [_ _ _ _ _ w1011 _]
              tunnel: w941 -> [_ w949 _ _ _ _ _]
              frame #0 {
                n547 = Build Array("Name", "Channel", "High limit", "Low limit") -> (w942:string[])
              }
              frame #1 {
                n548 = global read "Meas_global.vi" "LDA data"() -> (w947:enum16{"No LDA data", "Take LDA data"})
                n549 = case shown="\"Take LDA data\"" w947 {
                  tunnel: w949 -> [_ w960]
                  tunnel: [string[][] [] w957] -> w948
                  frame "No LDA data" {
                  }
                  frame "Take LDA data" {
                    n550 = global read "LDA_meas_global_1.vi" "Max Vel BSA1"() -> (w952:dbl)
                    n551 = global read "LDA_meas_global_1.vi" "Min Vel BSA1"() -> (w951:dbl)
                    n552 = global read "LDA_meas_global_1.vi" "Vel Comp BSA1"() -> (w961:string)
                    n553 = case shown="\"2D\"" w960 {
                      tunnel: [string[] [] w966] -> w958
                      frame "1D" {
                      }
                      frame "2D" {
                        n554 = global read "LDA_meas_global_2.vi" "Max Vel BSA2"() -> (w965:dbl)
                        n555 = global read "LDA_meas_global_2.vi" "Min Vel BSA2"() -> (w964:dbl)
                        n556 = global read "LDA_meas_global_2.vi" "Vel Comp BSA2"() -> (w967:string)
                        n557 = Format Into String(format string="%.1f m/s" ("Format String"), w964) -> (resulting string=w972:string)  [unwired: 2 in, 1 out]
                        n558 = Format Into String(format string="%.1f m/s" ("Format String"), w965) -> (resulting string=w971:string)  [unwired: 2 in, 1 out]
                        n559 = Build Array("LDA", w967, w971, w972) -> (w966:string[])
                      }
                    }
                    n560 = Format Into String(format string="%.1f m/s" ("Format String"), w951) -> (resulting string=w953:string)  [unwired: 2 in, 1 out]
                    n561 = Format Into String(format string="%.1f m/s" ("Format String"), w952) -> (resulting string=w954:string)  [unwired: 2 in, 1 out]
                    n562 = Build Array("LDA", w961, w954, w953) -> (w959:string[])
                    n563 = Build Array(w959, w958) -> (w957:string[][])
                  }
                }
              }
              frame #2 {
                n564 = global read "Meas_global.vi" "PWA Data"() -> (w974:T28)
                n565 = case shown="\"One Ch PWA\"" w974 {
                  tunnel: [string[][] [] w976] -> w973
                  frame "No PWA Data" {
                  }
                  frame "One Ch PWA" {
                    n566 = Build Array("PWA") -> (w977:string[])
                    n567 = Build Array(w977) -> (w976:string[][])
                  }
                }
              }
              frame #3 {
                n568 = global read "Meas_global.vi" "Ch & spans"() -> (w980:T25[])
                n569 = for {
                  tunnel: w980 -> [w991] mode=indexing
                  tunnel: [w987] -> w979 mode=indexing
                  n570 = Unbundle By Name(w991) -> ("Var name"=w990:string, "Ch No"=w989:i16, "high limit (10V)"=w984:sgl, "low limit (-10V)"=w983:sgl)
                  n571 = Format Into String(format string="%.1f Volts" ("Format String"), w984) -> (resulting string=w982:string)  [unwired: 2 in, 1 out]
                  n572 = Format Into String(format string="%.1f Volts" ("Format String"), w983) -> (resulting string=w981:string)  [unwired: 2 in, 1 out]
                  n573 = Number To Decimal String(number=w989) -> (decimal integer string=w988:string)  [unwired: 1 out]
                  n574 = Build Array(w990, w988, w982, w981) -> (w987:string[])
                }
              }
              frame #4 {
                n575 = global read "Meas_global.vi" "Analysis Info cluster"() -> (w1000:T19[])
                n576 = for {
                  tunnel: w1000 -> [w1010] mode=indexing
                  tunnel: [w1009] -> w998 mode=indexing
                  n577 = Unbundle By Name(w1010) -> ("Inst name"=w1009:string)
                }
                n578 = global read "Meas_global.vi" "correlate"() -> (w999:i32[][])
                n579 = for {
                  tunnel: w999 -> [w1005] mode=indexing
                  tunnel: w998 -> [w1004]
                  tunnel: "Correlating" -> [w1003]
                  tunnel: [w1001] -> w993 mode=indexing
                  n580 = for {
                    tunnel: w1005 -> [w1008] mode=indexing
                    tunnel: w1004 -> [w1007]
                    tunnel: [w1006] -> w1002 mode=indexing
                    n581 = Index Array(array=w1007, index=w1008) -> (element=w1006:string)
                  }
                  n582 = Build Array (concatenate)(w1003, w1002) -> (w1001:string[])
                }
                n583 = Initialize Array("", 5 ("Dimension Size")) -> (w994:string[])
                n584 = Build Array (concatenate)(w994, w993) -> (w992:string[][])
              }
              frame #5 {
                n585 = Build Array (concatenate)(w1016, w1015, w1011, w1014, w1012) -> (w1013:string[][])
                n586 = local write "Statistics"(w1013) -> ()
              }
              frame #6 {
                n587 = case shown="\"Take LDA data\"" w1025 {
                  tunnel: [string[] [] w1027] -> w1022
                  frame "No LDA data" {
                  }
                  frame "Take LDA data" {
                    n588 = global read "Meas_global.vi" "Synchronise with LDA"() -> (w1032:bool)
                    n589 = global read "Meas_global.vi" "Ch & spans"() -> (w1035:T25[])
                    n590 = Array Size(array=w1035) -> (size(s)=w1034:i32)
                    n591 = Greater Than 0?(x=w1034) -> (x > 0?=w1033:bool)
                    n592 = Compound Arithmetic op=AND(w1032, w1033) -> (w1031:bool)
                    n593 = Select(t="Synchronised with LDA", s=w1031, f="") -> (s? t:f=w1028:string)
                    n594 = Build Array(w1028) -> (w1027:string[])
                  }
                }
                n595 = global read "Meas_global.vi" "Continuous time trace?"() -> (w1017:bool)
                n596 = Select(t="Continuous Time Trace", s=w1017, f="") -> (s? t:f=w1021:string)
                n597 = Build Array (concatenate)(w1022, w1021) -> (w1020:string[])
                n598 = Build Array(w1020) -> (w1019:string[][])
                n599 = Transpose 2D Array(2D array=w1019) -> (transposed array=w1018:string[][])
                n600 = local write "Diagnostic info"(w1018) -> ()
              }
            }
          }
        }
      }
      frame #19 {
        n601 = local read "File"() -> (w1046:T5)
        n602 = Equal?(x=Setup."Run Program" ("setup"), y=w1047) -> (x = y?=w1044:bool)
        n603 = Not Equal?(x=w1046, y=Save_Data."Save No Data" ("File")) -> (x != y?=w1045:bool)
        n604 = global read "Meas_global.vi" "Repeat Measurement?"() -> (w1036:bool)
        n605 = Compound Arithmetic op=AND(invert w1036, w1044, w1045) -> (w1043:bool)
        n606 = Get Date/Time In Seconds() -> (seconds since 1Jan1904=w1040:timestamp)
        n607 = To Double Precision Float(number=w1040) -> (double precision float=w1038:dbl)
        n608 = local read "Setup filename"() -> (w1041:string)
        n609 = case shown="False" w1043 {
          tunnel: w1046 -> [_ _]
          tunnel: w1038 -> [w1050 w1083]
          tunnel: w1041 -> [w1049 w1082]
          tunnel: w1037 -> [w1048 w1081]
          frame True {
            n610 = stacked-sequence {
              seq-local: [_ w1054 _] -> [_ _ w1074]
              tunnel: w1050 -> [w1053 _ _]
              tunnel: w1049 -> [w1052 _ _]
              tunnel: w1048 -> [w1051 _ _]
              frame #0 {
                n611 = call "Write_Results_file.vi"("Experiment start time"=w1051, "Experiment End time"=w1053, "Setup filename"=w1052) -> ()  [unwired: 4 out]
              }
              frame #1 {
                w1059 = FALSE  # Empty list
                n612 = global read "Meas_global.vi" "Raw data file"() -> (w1058:path)
                n613 = global read "Trav_pos_global.vi" "Top level setup filename"() -> (w1056:path)
                n614 = global read "Meas_global.vi" "Start Time of experiment"() -> (w1055:dbl)
                n615 = Strip Path(path=w1058) -> (stripped path=w1054:path)  [unwired: 1 out]
                n616 = Empty String/Path?(string/path=w1056) -> (empty?=w1057:bool)
                n617 = case shown="False" w1057 {
                  tunnel: w1056 -> [w1073 _]
                  tunnel: w1054 -> [w1071 _]
                  tunnel: w1055 -> [w1069 _]
                  frame False {
                    n618 = call "Sec_to_date_filename.vi"("seconds"=w1069) -> ("Day"=w1068:string, "Time"=w1067:string)  [unwired: 2 out]
                    n619 = Format Into String(format string="Cmd_%s_%s.xls", w1068, w1067) -> (resulting string=w1065:string)  [unwired: 2 in, 1 out]
                    n620 = call "Fast_string_Replace.vi"("Replace match with:"="-", "Input String"=w1065, "regular expression"=":") -> ("Output String"=w1062:string)  [unwired: 2 out]
                    n621 = call "Fast_string_Replace.vi"("Replace match with:"="", "Input String"=w1062, "regular expression"=" ") -> ("Output String"=w1060:string)  [unwired: 2 out]
                    n622 = Build Path(base path=w1071, name or relative path=w1060) -> (appended path=w1070:path)
                    n623 = Copy(10:w1070, 11:w1073) -> ()  [unwired: 1 in, 5 out]
                  }
                  frame True {
                  }
                }
                n624 = call "Remember_RD_Folders.vi"("Empty list"=w1059, "Folders to Remember"=w1054) -> ()  [unwired: 1 out]
              }
              frame #2 {
                n625 = global read "Meas_global.vi" "LDA data"() -> (w1075:enum16{"No LDA data", "Take LDA data"})
                n626 = case shown="\"Take LDA data\"" w1075 {
                  tunnel: w1074 -> [_ w1079]
                  frame "No LDA data" {
                  }
                  frame "Take LDA data" {
                    w1077 = "LDA_Probe_Orientation.txt" ("name or relative path")
                    n627 = call "Setup_Filepath.vi"("Setup File Type"=Setup_Filetype."General", "Filename in"=w1077) -> ("Filename Out"=w1076:path)  [unwired: 1 out]
                    n628 = Build Path(base path=w1079, name or relative path=w1077) -> (appended path=w1080:path)
                    n629 = Copy(10:w1080, 11:w1076) -> ()  [unwired: 1 in, 5 out]
                  }
                }
              }
            }
          }
          frame False {
            n630 = global read "Meas_global.vi" "Raw data option"() -> (w1084:enum16{"Save raw data", "Raw data not saved"})
            n631 = case shown="\"Save raw data\"" w1084 {
              tunnel: w1081 -> [w1087 _]
              tunnel: w1083 -> [w1086 _]
              tunnel: w1082 -> [w1085 _]
              frame "Save raw data" {
                n632 = stacked-sequence {
                  tunnel: w1087 -> [_ w1096]
                  tunnel: w1086 -> [_ w1095]
                  tunnel: w1085 -> [_ w1093]
                  frame #0 {
                    n633 = global read "Meas_global.vi" "Current Block No"() -> (w1088:i32)
                    n634 = global write "Meas_global.vi" "Requested No of blocks"(w1088) -> ()
                  }
                  frame #1 {
                    n635 = call "Create_Raw_data_file.vi"("No of averages"=1, "End time"=w1095, "Start time"=w1096, "Setup filename"=w1093) -> ("Values"=w1091:string[][], "Column headers"=w1092:string[])  [unwired: 2 out]
                    n636 = Index Array(array=w1091, index (row)=0) -> (element=w1089:string[])  [unwired: 1 in]
                    n637 = global write "Dynamic_call_global.ph.vi" "Plug in values"(w1089) -> ()
                    n638 = global write "Dynamic_call_global.ph.vi" "Plug in titles"(w1092) -> ()
                  }
                }
              }
              frame "Raw data not saved" {
              }
            }
          }
        }
      }
      frame #20 {
        n639 = stacked-sequence {
          seq-local: [w1105 _ _] -> [_ w1112 _]
          seq-local: [w1102 _ _] -> [_ w1111 w1152]
          seq-local: [w1098 _ _] -> [_ _ w1151]
          tunnel: w1097 -> [w1110 _ _]
          frame #0 {
            n640 = global read "Meas_global.vi" "Raw data file"() -> (w1103:path)
            n641 = global read "Meas_global.vi" "Raw data option"() -> (w1109:enum16{"Save raw data", "Raw data not saved"})
            n642 = Equal?(x=Setup."Run Program" ("setup"), y=w1110) -> (x = y?=w1100:bool)
            n643 = Strip Path(path=w1103) -> (stripped path=w1099:path)  [unwired: 1 out]
            n644 = Equal?(x=w1109, y=enum16{"Save raw data", "Raw data not saved"}."Save raw data" ("Raw data option")) -> (x = y?=w1098:bool)
            n645 = Build Path(base path=w1099, name or relative path="VI_History.xls") -> (appended path=w1102:path)
            n646 = call "Does_file_exist_(simple).vi"("Pathname"=w1102) -> ("exists?"=w1107:bool)
            n647 = Not(x=w1107) -> (.not. x?=w1106:bool)
            n648 = Compound Arithmetic op=AND(w1106, w1100, w1098) -> (w1105:bool)
          }
          frame #1 {
            n649 = case shown="True" w1112 {
              tunnel: w1111 -> [_ w1113]
              frame False {
              }
              frame True {
                n650 = stacked-sequence {
                  tunnel: w1113 -> [w1119 w1127]
                  frame #0 {
                    w1116 = FALSE  # Lock File
                    n651 = global read "Meas_global.vi" "ProgRevisionInfo"() -> (w1115:string)
                    n652 = call "Characters_to_string.vi"("Characters to write"=w1115, "Label for characters"="Prog Revision info") -> ("Output string"=w1121:string)
                    n653 = call "Date_and_Time_to_string.vi"() -> ("Date and time (spreadsheet)"=w1122:string)
                    n654 = call "Get_mod_dates.vi"() -> ("error out"=w1120:errorcluster, "Output string"=w1117:string)  [unwired: 1 in, 3 out]
                    n655 = call "EnFlo_Error_Handler.vi"("error in (no error)"=w1120) -> ()  [unwired: 2 in, 3 out]
                    n656 = Concatenate Strings(w1122, w1121, w1117) -> (w1118:string)
                    n657 = call "Write_Characters_To_File.vi"("file path (dialog if empty)"=w1119, "character string"=w1118, "Lock File"=w1116) -> ()  [unwired: 2 in, 4 out]
                  }
                  frame #1 {
                    n658 = global read "Trav_pos_global.vi" "Traverses to Move"() -> (w1125:string[])
                    n659 = global read "Constants_global.vi" "Traverse folder"() -> (w1126:path)
                    n660 = Strip Path(path=w1127) -> (stripped path=w1124:path)  [unwired: 1 out]
                    n661 = for {
                      tunnel: w1126 -> [w1139]
                      tunnel: w1125 -> [w1135] mode=indexing
                      tunnel: w1124 -> [w1136]
                      tunnel: string[] ["Traverse_Preferences.txt", "Traverse_Setup.xls"] ("Traverses to Move") -> [w1128]
                      n662 = Build Path(base path=w1139, name or relative path=w1135) -> (appended path=w1131:path)
                      n663 = Build Path(base path=w1131, name or relative path="Trav_Space_Files" ("Substring")) -> (appended path=w1138:path)
                      n664 = Build Path(base path=w1138, name or relative path="Selected_Filename.txt" ("Substring")) -> (appended path=w1143:path)
                      n665 = call "Create_directory_path.vi"("Path name"=w1143) -> ("Path name Out"=w1142:path)  [unwired: 2 in, 1 out]
                      n666 = Build Path(base path=w1136, name or relative path=w1135) -> (appended path=w1130:path)
                      n667 = for {
                        tunnel: w1131 -> [w1150]
                        tunnel: w1130 -> [w1148]
                        tunnel: w1128 -> [w1146] mode=indexing
                        n668 = Build Path(base path=w1150, name or relative path=w1146) -> (appended path=w1149:path)
                        n669 = Build Path(base path=w1148, name or relative path=w1146) -> (appended path=w1145:path)
                        n670 = call "Create_directory_path.vi"("Path name"=w1145) -> ("Path name Out"=w1144:path)  [unwired: 2 in, 1 out]
                        n671 = Copy(9:TRUE ("overwrite (F)"), 10:w1144, 11:w1149) -> ()  [unwired: 2 in, 3 out]
                      }
                      n672 = call "Read_File_Simple.vi"("Filename"=w1142) -> ("string"=w1133:string)  [unwired: 2 in, 7 out]
                      n673 = Build Path(base path=w1130, name or relative path=w1133) -> (appended path=w1134:path)
                      n674 = Build Path(base path=w1138, name or relative path=w1133) -> (appended path=w1137:path)
                      n675 = call "Create_directory_path.vi"("Path name"=w1134) -> ("Path name Out"=w1132:path)  [unwired: 2 in, 1 out]
                      n676 = Copy(9:TRUE ("overwrite (F)"), 10:w1132, 11:w1137) -> ()  [unwired: 2 in, 3 out]
                    }
                  }
                }
              }
            }
          }
          frame #2 {
            n677 = case shown="True" w1151 {
              tunnel: w1152 -> [_ w1159]
              frame False {
              }
              frame True {
                n678 = Strip Path(path=w1159) -> (stripped path=w1158:path)  [unwired: 1 out]
                n679 = local read "Setup filename"() -> (w1154:string)
                n680 = Build Path(base path=w1158, name or relative path="Measurement_Setups") -> (appended path=w1155:path)
                n681 = Build Path(base path=w1155, name or relative path=w1154) -> (appended path=w1153:path)
                n682 = call "Does_file_exist_(simple).vi"("Pathname"=w1153) -> ("exists?"=w1157:bool)
                n683 = case shown="False" w1157 {
                  tunnel: w1153 -> [w1161 _]
                  tunnel: w1154 -> [w1162 _]
                  frame False {
                    n684 = call "Create_directory_path.vi"("Path name"=w1161) -> ("Path name Out"=w1160:path)  [unwired: 2 in, 1 out]
                    n685 = call "Setup_Filepath.vi"("Setup File Type"=Setup_Filetype."Measurement Setups", "Filename in"=w1162) -> ("Filename Out"=w1163:path)  [unwired: 1 out]
                    n686 = Copy(9:TRUE ("overwrite (F)"), 10:w1160, 11:w1163) -> ()  [unwired: 2 in, 3 out]
                  }
                  frame True {
                  }
                }
              }
            }
          }
        }
      }
      frame #21 {
        n687 = local read "Correlate?"() -> (w1170:T9)
        n688 = case shown="\"Run Program\"" w1167 {
          tunnel: w1167 -> [w1172 _ _ _]
          tunnel: [w1172 w1185 w1186 w1187] -> w1166
          frame "Run Program" {
            n689 = global read "Meas_global.vi" "Analysis Info cluster"() -> (w1171:T19[])
            n690 = for {
              tunnel: w1171 -> [w1183] mode=indexing
              stop <- w1173 stop-if-true
              w1180 = "Pitot ("
              n691 = Unbundle By Name(w1183) -> ("U"=w1174:dbl, "Inst name"=w1179:string)
              n692 = String Length(string=w1180) -> (length=w1182:i32)
              n693 = String Subset(string=w1179, length (rest)=w1182) -> (substring=w1181:string)  [unwired: 1 out]
              n694 = Equal?(x=w1181, y=w1180) -> (x = y?=w1176:bool)
              n695 = call "Match_Pat_Case_In.vi"("String to match"="ref", "String"=w1179) -> ("offset past match"=w1177:i32)  [unwired: 1 in, 3 out]
              n696 = Greater Or Equal To 0?(x=w1177) -> (x >= 0?=w1175:bool)
              n697 = And(x=w1175, y=w1176) -> (x .and. y?=w1173:bool)
              n698 = case shown="True" w1173 {
                tunnel: w1174 -> [_ w1184]
                frame False {
                }
                frame True {
                  n699 = call "Log_Reference_Velocity.vi"("Measured Velocity"=w1184) -> ()  [unwired: 1 out]
                }
              }
            }
          }
          frame "Show Setup" {
            w1185 = Setup."Run Program"  # setup
          }
          frame "Save Current Setup" {
            w1186 = Setup."Run Program"  # setup
          }
          frame "Setup Front Panel" {
            w1187 = Setup."Run Program"  # setup
          }
        }
        n700 = case shown="\"Show correlation panel\"" w1170 {
          tunnel: [T9."Cross correlation off" T9."Correlate without activating panel" T9."Correlate without activating panel"] -> w1169
          frame "Cross correlation off" {
          }
          frame "Show correlation panel" {
          }
          frame "Correlate without activating panel" {
          }
        }
        n701 = local write "Correlate?"(w1169) -> ()
        n702 = global write "Meas_global.vi" "Remote control"(FALSE ("Remote control")) -> ()
        n703 = call "Program_Active.vi"() -> ()  [unwired: 1 in]
        n704 = local write "setup"(w1166) -> ()
      }
      frame #22 {
        w1196 = FALSE  # Dialog Box (T)
        n705 = global read "Meas_global.vi" "Post Process"() -> (w1191:T2)
        n706 = case shown="\"Take New Data\"" w1191 {
          frame "Take New Data" {
            n707 = global read "Meas_global.vi" "Requested Sampling rate"() -> (w1219:dbl)
            n708 = global read "Meas_global.vi" "Analysis Info cluster"() -> (w1215:T19[])
            n709 = Divide(x=w1219, y=10.0) -> (x/y=w1216:dbl)
            n710 = Max & Min(x=w1216, y=100.0) -> (min(x,y)=w1214:dbl)  [unwired: 1 out]
            n711 = for {
              tunnel: w1215 -> [w1250] mode=indexing
              tunnel: w1214 -> [w1245]
              tunnel: [w1243] -> w1211 mode=indexing if=w1239
              tunnel: [w1240] -> w1202 mode=indexing if=w1241
              tunnel: [w1240] -> w1200 mode=indexing if=w1239
              n712 = Unbundle By Name(w1250) -> ("Inst name"=w1244:string, "Av Sampling Rate"=w1243:dbl, "Inst type"=w1249:T14)
              n713 = Equal?(x=w1249, y=Inst_type."LDA Vel" ("Inst type")) -> (x = y?=w1239:bool)
              n714 = Greater Than 0?(x=w1243) -> (x > 0?=w1246:bool)
              n715 = Less?(x=w1243, y=w1245) -> (x < y?=w1247:bool)
              n716 = Compound Arithmetic op=AND(w1247, w1246, w1239) -> (w1241:bool)
              n717 = Format Into String(format string="The %s currently has a data rate of %d Hz\n", w1244, w1243) -> (resulting string=w1240:string)  [unwired: 2 in, 1 out]
            }
            n718 = Array Max & Min(array=w1211) -> (max value=w1209:dbl, min value=w1208:dbl)  [unwired: 2 out]
            n719 = Array Size(array=w1211) -> (size(s)=w1210:i32)
            n720 = Concatenate Strings(w1200) -> (w1199:string)
            n721 = Concatenate Strings(w1202) -> (w1201:string)
            n722 = Empty String/Path?(string/path=w1201) -> (empty?=w1213:bool)
            n723 = case shown="False" w1213 {
              tunnel: [w1230 FALSE] -> w1212
              frame False {
                n724 = global read "Preference_global.vi" "Rig Setup"() -> (w1236:string)
                n725 = Concatenate Strings("Status:of:", w1236) -> (w1235:string)
                n726 = Build Array(w1235) -> (w1234:string[])
                n727 = call "Get_Current_Scan_client.vi"("ADAM Ch Names"=w1234) -> ("Numerical Values"=w1233:dbl[])  [unwired: 1 in, 2 out]
                n728 = Index Array(array=w1233) -> (element=w1232:dbl)  [unwired: 1 in]
                n729 = Equal?(x=2.0, y=w1232) -> (x = y?=w1230:bool)
              }
              frame True {
              }
            }
            n730 = case shown="True" w1212 {
              tunnel: w1201 -> [_ w1225]
              frame False {
              }
              frame True {
                w1228 = FALSE  # Dialog Box (T)
                n731 = Bundle By Name(cluster=errorcluster {"status"=TRUE, "code"=0, "source"=""} ("error in (no error)"), "source"=w1225) -> (w1227:errorcluster)
                n732 = call "EnFlo_Error_Handler.vi"("error in (no error)"=w1227, "Error Type"="Low LDA Sampling Rate", "Dialog Box (T)"=w1228) -> ()  [unwired: 3 out]
              }
            }
            n733 = Greater Than 0?(x=w1210) -> (x > 0?=w1205:bool)
            n734 = Divide(x=w1209, y=w1208) -> (x/y=w1203:dbl)
            n735 = Greater?(x=w1203, y=4.0) -> (0:w1206:bool)
            n736 = And(x=w1205, y=w1206) -> (x .and. y?=w1204:bool)
            n737 = case shown="True" w1204 {
              tunnel: w1199 -> [_ w1220]
              frame False {
              }
              frame True {
                w1223 = FALSE  # Dialog Box (T)
                n738 = Bundle By Name(cluster=errorcluster {"status"=TRUE, "code"=0, "source"=""} ("error in (no error)"), "source"=w1220) -> (w1222:errorcluster)
                n739 = call "EnFlo_Error_Handler.vi"("error in (no error)"=w1222, "Error Type"="LDA Data rate ratio greater than 4", "Dialog Box (T)"=w1223) -> ()  [unwired: 3 out]
              }
            }
          }
          frame "Post Process Raw Data File" {
          }
        }
        n740 = global read "Meas_global.vi" "Over/Under string"() -> (w1194:string)
        n741 = Empty String/Path?(string/path=w1194) -> (empty?=w1193:bool)
        n742 = Not(x=w1193) -> (.not. x?=w1192:bool)
        n743 = Bundle By Name(cluster=errorcluster {"status"=FALSE, "code"=0, "source"=""} ("error in (no error)"), "source"=w1194, "status"=w1192) -> (w1197:errorcluster)
        n744 = call "EnFlo_Error_Handler.vi"("error in (no error)"=w1197, "Error Type"="Signal Clipping", "Dialog Box (T)"=w1196) -> ()  [unwired: 3 out]
      }
      frame #23 {
        w1254 = string[] [] ("Per Block Plug Ins Extra")
        n745 = Empty String/Path?(string/path=w1251) -> (empty?=w1257:bool)
        n746 = global read "Dynamic_call_global.ph.vi" "Final Plug Ins"() -> (w1258:string[])
        n747 = case shown="True" w1257 {
          tunnel: w1251 -> [w1269 _]
          frame False {
            n748 = local read "Comments"() -> (w1268:string)
            n749 = call "Fast_string_Replace.vi"("Replace match with:"="", "Input String"=w1268, "regular expression"=w1269) -> ("Output String"=w1267:string)  [unwired: 2 out]
            n750 = local write "Comments"(w1267) -> ()
          }
          frame True {
          }
        }
        n751 = call "Plug_in_Directories.vi"() -> ("Final"=w1255:path)  [unwired: 3 out]
        n752 = for {
          tunnel: w1258 -> [w1272] mode=indexing
          tunnel: w1255 -> [w1271]
          w1275 = FALSE  # Dialog Box (T)
          n753 = Build Path(base path=w1271, name or relative path=w1272) -> (appended path=w1270:path)
          n754 = global read "Dynamic_call_global.ph.vi" "Plug in"() -> (w1280:refnum<vi>)
          n755 = Open VI Reference(type specifier VI Refnum (for type only)=w1280, vi path=w1270) -> (vi reference=w1279:refnum<vi>, error out=w1278:errorcluster)  [unwired: 2 in, 2 out]
          n756 = call-by-ref "?"(reference=w1279, error in=w1278) -> (reference out=w1276:refnum<vi>, error out=w1277:errorcluster)  [unwired: 6 in, 2 out]
          n757 = Close Reference(reference=w1276, error in (no error)=w1277) -> (error out=w1273:errorcluster)
          n758 = call "EnFlo_Error_Handler.vi"("error in (no error)"=w1273, "Error Type"="Running Final Plug In", "Dialog Box (T)"=w1275) -> ()  [unwired: 3 out]
        }
        n759 = global read "Meas_global.vi" "Repeat Measurement?"() -> (w1256:bool)
        n760 = case shown="True" w1256 {
          tunnel: w1253 -> [_ w1265]
          tunnel: [FALSE w1260] -> w1252
          frame False {
          }
          frame True {
            n761 = global read "Meas_global.vi" "Post Process"() -> (w1263:T2)
            n762 = Equal To 0?(x=w1265) -> (x = 0?=w1261:bool)
            n763 = Equal?(x=w1263, y=Post_Process."Post Process Raw Data File" ("Post Process")) -> (x = y?=w1262:bool)
            n764 = And(x=w1262, y=w1261) -> (x .and. y?=w1260:bool)
          }
        }
        n765 = global write "Dynamic_call_global.ph.vi" "Per Block Plug Ins Extra"(w1254) -> ()
        n766 = global write "Dynamic_call_global.ph.vi" "Initial Plug Ins Extra"(w1254) -> ()
      }
      frame #24 {
        n767 = global read "Meas_global.vi" "Post Process"() -> (w1287:T2)
        n768 = local read "stop"() -> (w1293:bool)
        n769 = Equal?(x=w1288, y=Setup."Run Program" ("setup")) -> (x = y?=w1284:bool)
        n770 = Equal?(x=w1287, y=Post_Process."Take New Data" ("Post Process")) -> (x = y?=w1285:bool)
        n771 = And(x=w1284, y=w1285) -> (x .and. y?=w1283:bool)
        n772 = case shown="False" w1293 {
          tunnel: [Multi_Run_Status."Continue" ("Status Out") Multi_Run_Status."Terminate Run" ("Status Out")] -> w1291
          frame False {
          }
          frame True {
            n773 = local write "stop"(FALSE) -> ()
          }
        }
        n774 = case shown="True" w1283 {
          tunnel: w1291 -> [w1294 w1297]
          tunnel: [w1294 w1299] -> w1290
          frame False {
          }
          frame True {
            n775 = local read "Raw data file"() -> (w1298:path)
            n776 = Path to Array of Strings(0:w1298) -> (2:w1300:string[])  [unwired: 1 out]
            n777 = Index Array(array=w1300, index=0 ("Index")) -> (element=w1296:string)
            n778 = Build Array(w1296) -> (w1295:string[])
            n779 = for {
              tunnel: w1295 -> [w1304] mode=indexing
              shift-right: [w1302] -> w1299
              shift-left: w1297 -> [w1303]
              n780 = call "Warn_on_low_HD_space.vi"("Status In"=w1303, "HD name"=w1304) -> ("Status Out"=w1302:T1)  [unwired: 6 out]
            }
          }
        }
        "Status Out" <- w1290
        n781 = global write "Trav_pos_global.vi" "Dummy Measurement?"(FALSE ("Dummy Measurement?")) -> ()
        n782 = global write "Plug_in_data_global.vi" "Server Channels to log"(string[] [] ("Server Channels to log")) -> ()
        n783 = global write "Meas_global.vi" "Extra Comments"("") -> ()
      }
    }
  }
